vi "HOST_1712.vi"() -> ()   [LabVIEW 2018]
uses:
  <vilib>/userdefined/High Color/nirio_resource_hc.ctl
  <instrlib>/niDCPower/nidcpower.llb/niDCPower Measurement Type.ctl
  <vilib>/FPGAPlugInAG/PXI-7953R/niLvFpga_Open_PXI-7953R.vi
  <vilib>/rvi/interface/common/dynamic/niFpgaDynamicAddResources.vi
  <vilib>/FPGAPlugInAG/Dynamic/niLvFpga_Reset_Dynamic.vi
  <vilib>/FPGAPlugInAG/Dynamic/niLvFpga_Run_Dynamic.vi
  <vilib>/Utility/error.llb/Error Cluster From Error Code.vi
  <vilib>/rvi/errors/niLvFpgaAdjustHostInterfaceError.vi
  <vilib>/FPGAPlugInAG/Dynamic/niLvFpga_Close_Dynamic.vi
  <vilib>/rvi/interface/nirviOpenFPGA/nirviOpenFPGA.xnode
  FPGA Bitfiles/1712_FPGATarget_TARGET1712_0YSosfiRP6w.lvbitx
  <vilib>/rvi/interface/nirviMethod/nirviMethod.xnode
  <vilib>/rvi/interface/nirviReadWriteControl/nirviReadWriteControl.xnode
  <vilib>/rvi/interface/nirviCloseFPGA/nirviCloseFPGA.xnode
  NiFpgaLv.dll
  <vilib>/rvi/interface/Simulation/niFpgaSimulationCallBeginRW.vi
  <vilib>/FPGAPlugInAG/Dynamic/niLvFpga_ReadFifo_Dynamic.vi
  <vilib>/rvi/errors/niLvFpgaMergeErrorWithErrorCode.vi
  <vilib>/Analysis/NI_AALPro.lvlib
panel:
  in  "Включаем автоматом?":bool
  out "VDD":i32
  out "PS":i32
  out "ADC":i32
  out "STAB":i32
  out "-15":i32
  out "4V":i32
  out "RD":i32
  out "PH":i32
  out "1V":i32
  out "БД":i32
  out "Эфф. по верт.":dbl
  out "Эфф. по гор.":dbl
  in  "Частота?":enum16{"MIN", "MAX"}(ring)
  out "СКО выхода от выхода":cluster{dbl[], dbl[]}(graph)={[6201.177706552707, 7595.434558404559, 8732.705797720797, 10087.72774928775, 11406.968846153846, 12631.295284900283, 14025.915, 15297.925598290598, 16480.01816239316, 17633.976495726496, 18869.50398860399, 20178.697706552706, 21306.84829059829, 22549.05603988604, 23809.401296296295, 24777.888917378918, 25884.07384615385, 27016.14232193732, 28208.568333333336, 29233.02923076923, 30354.480085470084, 31398.67948717949, 32328.064900284902, 32988.004458689466, 33587.57784900285, 34215.26438746438, 34782.93656695157, 35292.22700854701, 35768.959216524214, 36186.2800997151, 36566.8903988604, 36910.31642450143, 37239.01190883191, 37548.589829059834, 37829.74592592593, 38094.46146723647, 38321.56247863248, 38509.039344729346, 38634.09653846154, 38688.332564102566], [1408.2462455537227, 1276.6738405632493, 1421.2168940467238, 1726.6350596022562, 1769.1841993647113, 2160.503960124062, 2252.79189873594, 2374.7481159835115, 2690.694572350192, 2422.9048269586224, 2894.1814706198184, 3106.4349457710996, 3064.1792073843126, 3174.8802855895538, 3734.0833095929265, 4280.53840903318, 5096.146959046002, 5242.581747893684, 5382.248367652099, 5356.227733206448, 5575.580587757664, 5438.475052707056, 5246.7833296664485, 6997.312064633342, 6766.519928378316, 6762.928043979101, 6915.84030212127, 7792.281989480644, 8321.967233913709, 8296.431780392239, 10049.627295205792, 10386.237369576253, 10672.701676543498, 9213.355750556748, 9682.971733830318, 9250.473172388141, 10253.422148829253, 9607.6837198, 10679.138619744117, 10335.552449343717]}
  in  "Усреднение":i32=2
  out "Ке":dbl
  in  "Какая фотка?":string
  in  "НЕПРЕРЫВНО":bool
  out "СКО":dbl
  in  "ISO":dbl=1.0
  out "Среднее":dbl
  out "Фотонная калибровка":cluster{dbl[], dbl[]}(graph)={[6201.177706552707, 7595.434558404559, 8732.705797720797, 10087.72774928775, 11406.968846153846, 12631.295284900283, 14025.915, 15297.925598290598, 16480.01816239316, 17633.976495726496, 18869.50398860399, 20178.697706552706, 21306.84829059829, 22549.05603988604, 23809.401296296295, 24777.888917378918, 25884.07384615385, 27016.14232193732, 28208.568333333336, 29233.02923076923, 30354.480085470084, 31398.67948717949, 32328.064900284902, 32988.004458689466, 33587.57784900285, 34215.26438746438, 34782.93656695157, 35292.22700854701, 35768.959216524214, 36186.2800997151, 36566.8903988604, 36910.31642450143, 37239.01190883191, 37548.589829059834, 37829.74592592593, 38094.46146723647, 38321.56247863248, 38509.039344729346, 38634.09653846154, 38688.332564102566], [1408.2462455537227, 1276.6738405632493, 1421.2168940467238, 1726.6350596022562, 1769.1841993647113, 2160.503960124062, 2252.79189873594, 2374.7481159835115, 2690.694572350192, 2422.9048269586224, 2894.1814706198184, 3106.4349457710996, 3064.1792073843126, 3174.8802855895538, 3734.0833095929265, 4280.53840903318, 5096.146959046002, 5242.581747893684, 5382.248367652099, 5356.227733206448, 5575.580587757664, 5438.475052707056, 5246.7833296664485, 6997.312064633342, 6766.519928378316, 6762.928043979101, 6915.84030212127, 7792.281989480644, 8321.967233913709, 8296.431780392239, 10049.627295205792, 10386.237369576253, 10672.701676543498, 9213.355750556748, 9682.971733830318, 9250.473172388141, 10253.422148829253, 9607.6837198, 10679.138619744117, 10335.552449343717]}
  out "Usat, В":dbl
  out "Ssat, АЦП":dbl
  out "Коэффициент наклона":dbl
  out "Светосигнальная":cluster{u8, "ДИСКРЕТ, мс":u8, dbl[]}(graph)={1, "ДИСКРЕТ, мс"=4, [6201.177706552707, 7595.434558404559, 8732.705797720797, 10087.72774928775, 11406.968846153846, 12631.295284900283, 14025.915, 15297.925598290598, 16480.01816239316, 17633.976495726496, 18869.50398860399, 20178.697706552706, 21306.84829059829, 22549.05603988604, 23809.401296296295, 24777.888917378918, 25884.07384615385, 27016.14232193732, 28208.568333333336, 29233.02923076923, 30354.480085470084, 31398.67948717949, 32328.064900284902, 32988.004458689466, 33587.57784900285, 34215.26438746438, 34782.93656695157, 35292.22700854701, 35768.959216524214, 36186.2800997151, 36566.8903988604, 36910.31642450143, 37239.01190883191, 37548.589829059834, 37829.74592592593, 38094.46146723647, 38321.56247863248, 38509.039344729346, 38634.09653846154, 38688.332564102566]}
  in  "Между кадрами, мс":u8=1
  in  "Кол-во итераций":i32=40
  in  "ПРИМЕЧАНИЕ":string
  in  "Frames":path=path "C:/VPL/LabView_PRJ/DOZOR/1712/FRAMES"
  in  "ДИСКРЕТ, мс":u8=4
  out "FRAME_OK":bool
  in  "Расчет":bool
  in  "Какой канал?":enum16{"OUT1", "OUT2", "OUT4"}(ring)
  in  "+/- OUT2":enum16{"-", "+"}(ring)=enum."+"
  in  "Смещение, до 300_OUT2":dbl
  in  "Усиление (до 6)_OUT2":u8=1
  in  "Запись Кадра":bool
  out "АЦП прошит!":bool
  in  "Усиление (до 6)_OUT4":u8=1
  in  "+/- OUT4":enum16{"-", "+"}(ring)=enum."+"
  in  "Смещение, до 300_OUT4":dbl
  out "Image":T1(plugin-control)
  in  "文韧 世男!":bool
  in  "HIGH":u8=22
  in  "LOW":u8=9
  in  "8":u8=24
  in  "HOR":u16=465
  in  "PH1_1":u8=5
  in  "PH1_2":u8=17
  in  "PH2_1":u8=5
  in  "PH2_2":u8=17
  in  "RG1":u8=5
  in  "RG_2":u8=8
  in  "ADC_1":u8=9
  in  "ADC_2":u8=22
  in  "CDS2_1":u8=5
  in  "CDS2_2":u8=18
  in  "CDS1_1":u8=9
  in  "CDS1_2":u8=14
  in  "PS41_2":u16=710
  in  "PS41_1":u16=30
  in  "PS3_2":u16=843
  in  "PS3_1":u16=435
  in  "PS21_2":u16=573
  in  "PS21_1":u16=165
  in  "PS1_1":u16=300
  in  "PS1_2":u16=980
  in  "1163":u16=1163
  in  "Строка триггер":u16=100
  in  "Сколько строк?":i32=270
  in  "Усиление (до 6)_OUT1":u8=1
  in  "Смещение, до 300_OUT1":dbl
  in  "+/- OUT1":enum16{"-", "+"}(ring)=enum."+"
  in  "2/4 V":enum16{"2V", "4V"}(ring)
  in  "3CH/1CH":enum16{"3CH", "1CH"}(ring)=enum."1CH"
  out "Configuration":bool[](array[boolean])=[FALSE, FALSE, FALSE, TRUE, TRUE, FALSE, TRUE, FALSE, FALSE]
  out "PS":bool
  out "VDD":bool
  out "1V":bool
  out "PH":bool
  out "RD":bool
  out "4V":bool
  out "-15":bool
  in  "0,005":dbl=0.005 format="%#_13g"
  out "STAB":bool
  out "ADC":bool
  in  "Прошить АЦП":bool
  in  "PS_LOW, V":dbl=-8.0 caption="voltage level" format="%_6p"
  in  "PS_LOW_curlim":dbl=0.1 caption="current limit" format="%_6p"
  out "PS_LOW_cur":dbl caption="measurement" format="%_6g"
  in  "ADC, V":dbl=6.0 caption="voltage level" format="%_6p"
  in  "RD, V":dbl=13.0 caption="voltage level" format="%_6p"
  in  "PH_LOW, V":dbl=-3.5 caption="voltage level" format="%_6p"
  in  "VDD, V":dbl=17.0 caption="voltage level" format="%_6p"
  in  "ADC_curlim":dbl=0.2 caption="current limit" format="%_6p"
  in  "STAB_curlim":dbl=0.10000000000000003 caption="current limit" format="%_6p"
  in  "RD_curlim":dbl=0.1 caption="current limit" format="%_6p"
  in  "PH_LOW_curlim":dbl=0.1 caption="current limit" format="%_6p"
  in  "1V_curlim":dbl=0.1 caption="current limit" format="%_6p"
  in  "VDD_curlim":dbl=0.1 caption="current limit" format="%_6p"
  out "ADC_cur":dbl caption="measurement" format="%_6g"
  out "STAB_cur":dbl caption="measurement" format="%_6g"
  out "RD_cur":dbl caption="measurement" format="%_6g"
  out "PH_LOW_cur":dbl caption="measurement" format="%_6g"
  out "1V_cur":dbl caption="measurement" format="%_6g"
  out "VDD_cur":dbl caption="measurement" format="%_6g"
  in  "STAB, V":dbl=15.0 caption="voltage level" format="%_6p"
  in  "1V":dbl=1.0 caption="voltage level" format="%_6p"
  in  "4V":dbl=4.0 caption="voltage level" format="%_6p"
  in  "4V_curlim":dbl=0.1 caption="current limit" format="%_6p"
  out "4V_cur":dbl caption="measurement" format="%_6g"
  in  "-15_curlim":dbl=0.1 caption="current limit" format="%_6p"
  out "-15_cur":dbl caption="measurement" format="%_6g"
  in  "-15, V":dbl=-15.0 caption="voltage level" format="%_6p"
  in  "2":refnum<k15>="PXI1Slot4" caption="instrument handle"
  in  "0":refnum<k15>="PXI1Slot2" caption="instrument handle"
  in  "1":refnum<k15>="PXI1Slot3" caption="instrument handle"
  in  "resource name":T2="PXI1Slot5"
  in  "LOGS":path=path "C:/VPL/LabView_PRJ/DOZOR/1712/LOGS"
  in  "Линейки":bool
  in  "Питание":bool
  in  "Стоп":bool
  out "Номер образца":string="1"
  out "OUT":cluster{u16, u16, u16, u16}[][](array[cluster])
  out "FRAME":u16[][](array[numeric])
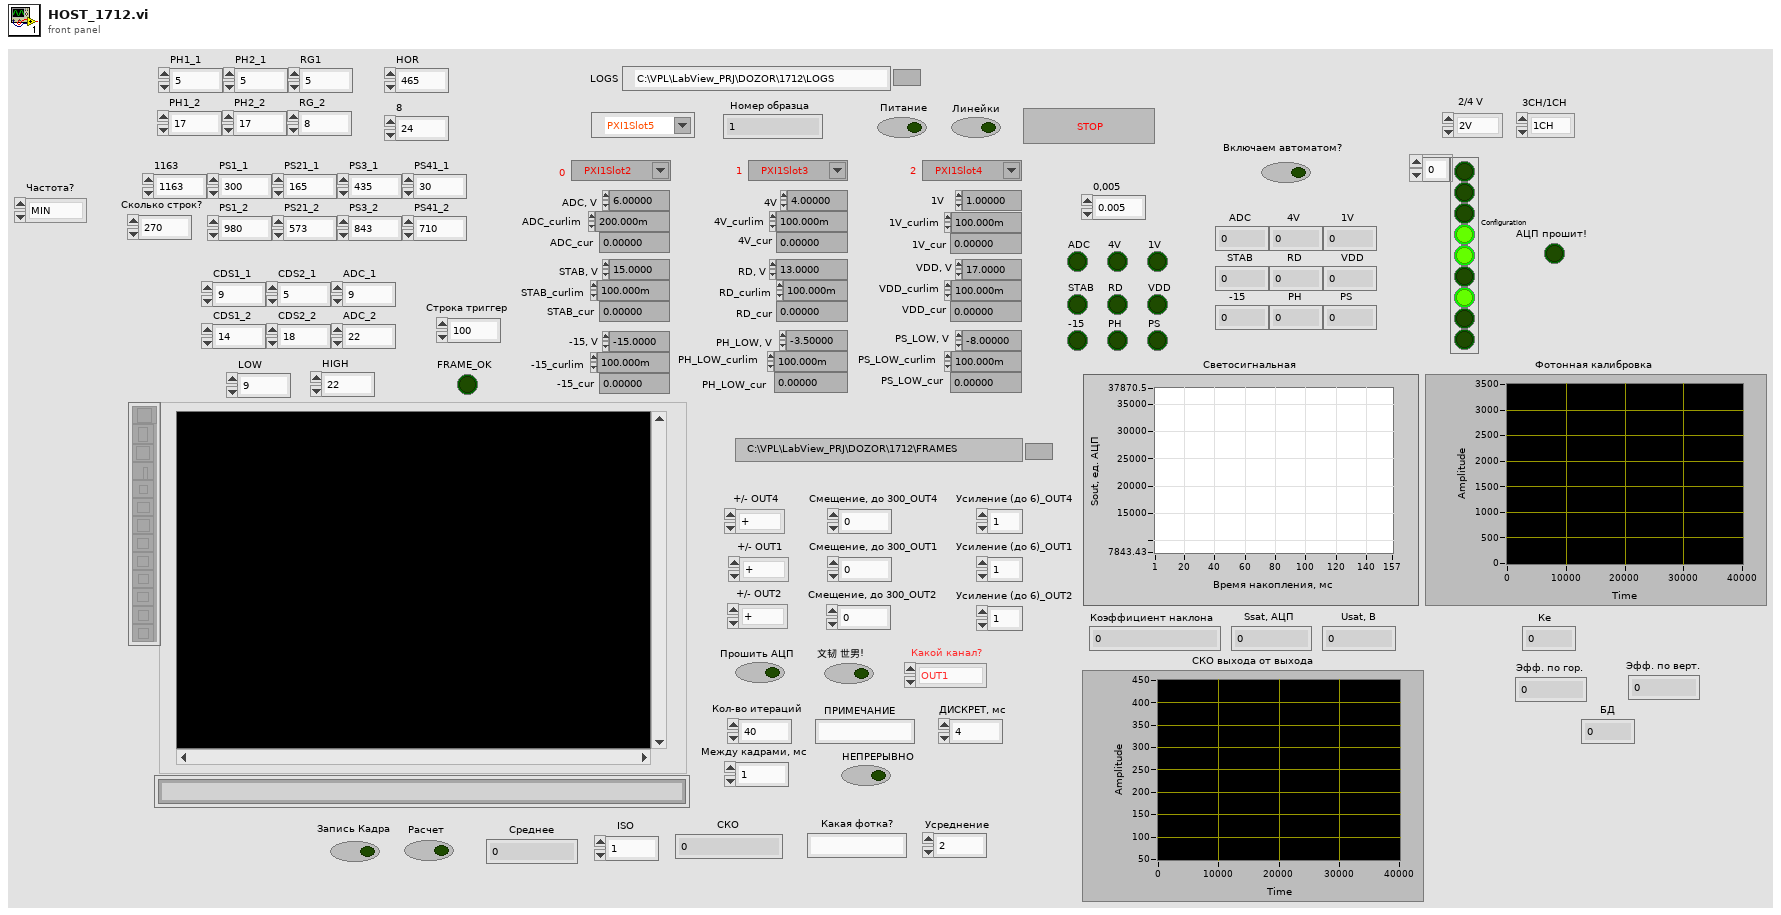
[diagram p1: front panel]
types:
  T1 = typedef "IMAQ Image.ctl" = refnum<image>
  T2 = typedef "nirio_resource_hc.ctl" = tag
  T3 = enum16{"open", "replace", "create", "open or create", "replace or create", "replace or create with confirmation"}
  T4 = typedef "niDCPower Measurement Type.ctl" = i32
  T5 = typedef "Image Type" = u32
  T6 = enum16{"Configuration", "MUX", "RED PGA", "GREEN PGA", "BLUE PGA", "RED OFF", "GREEN OFF", "BLUE OFF"}
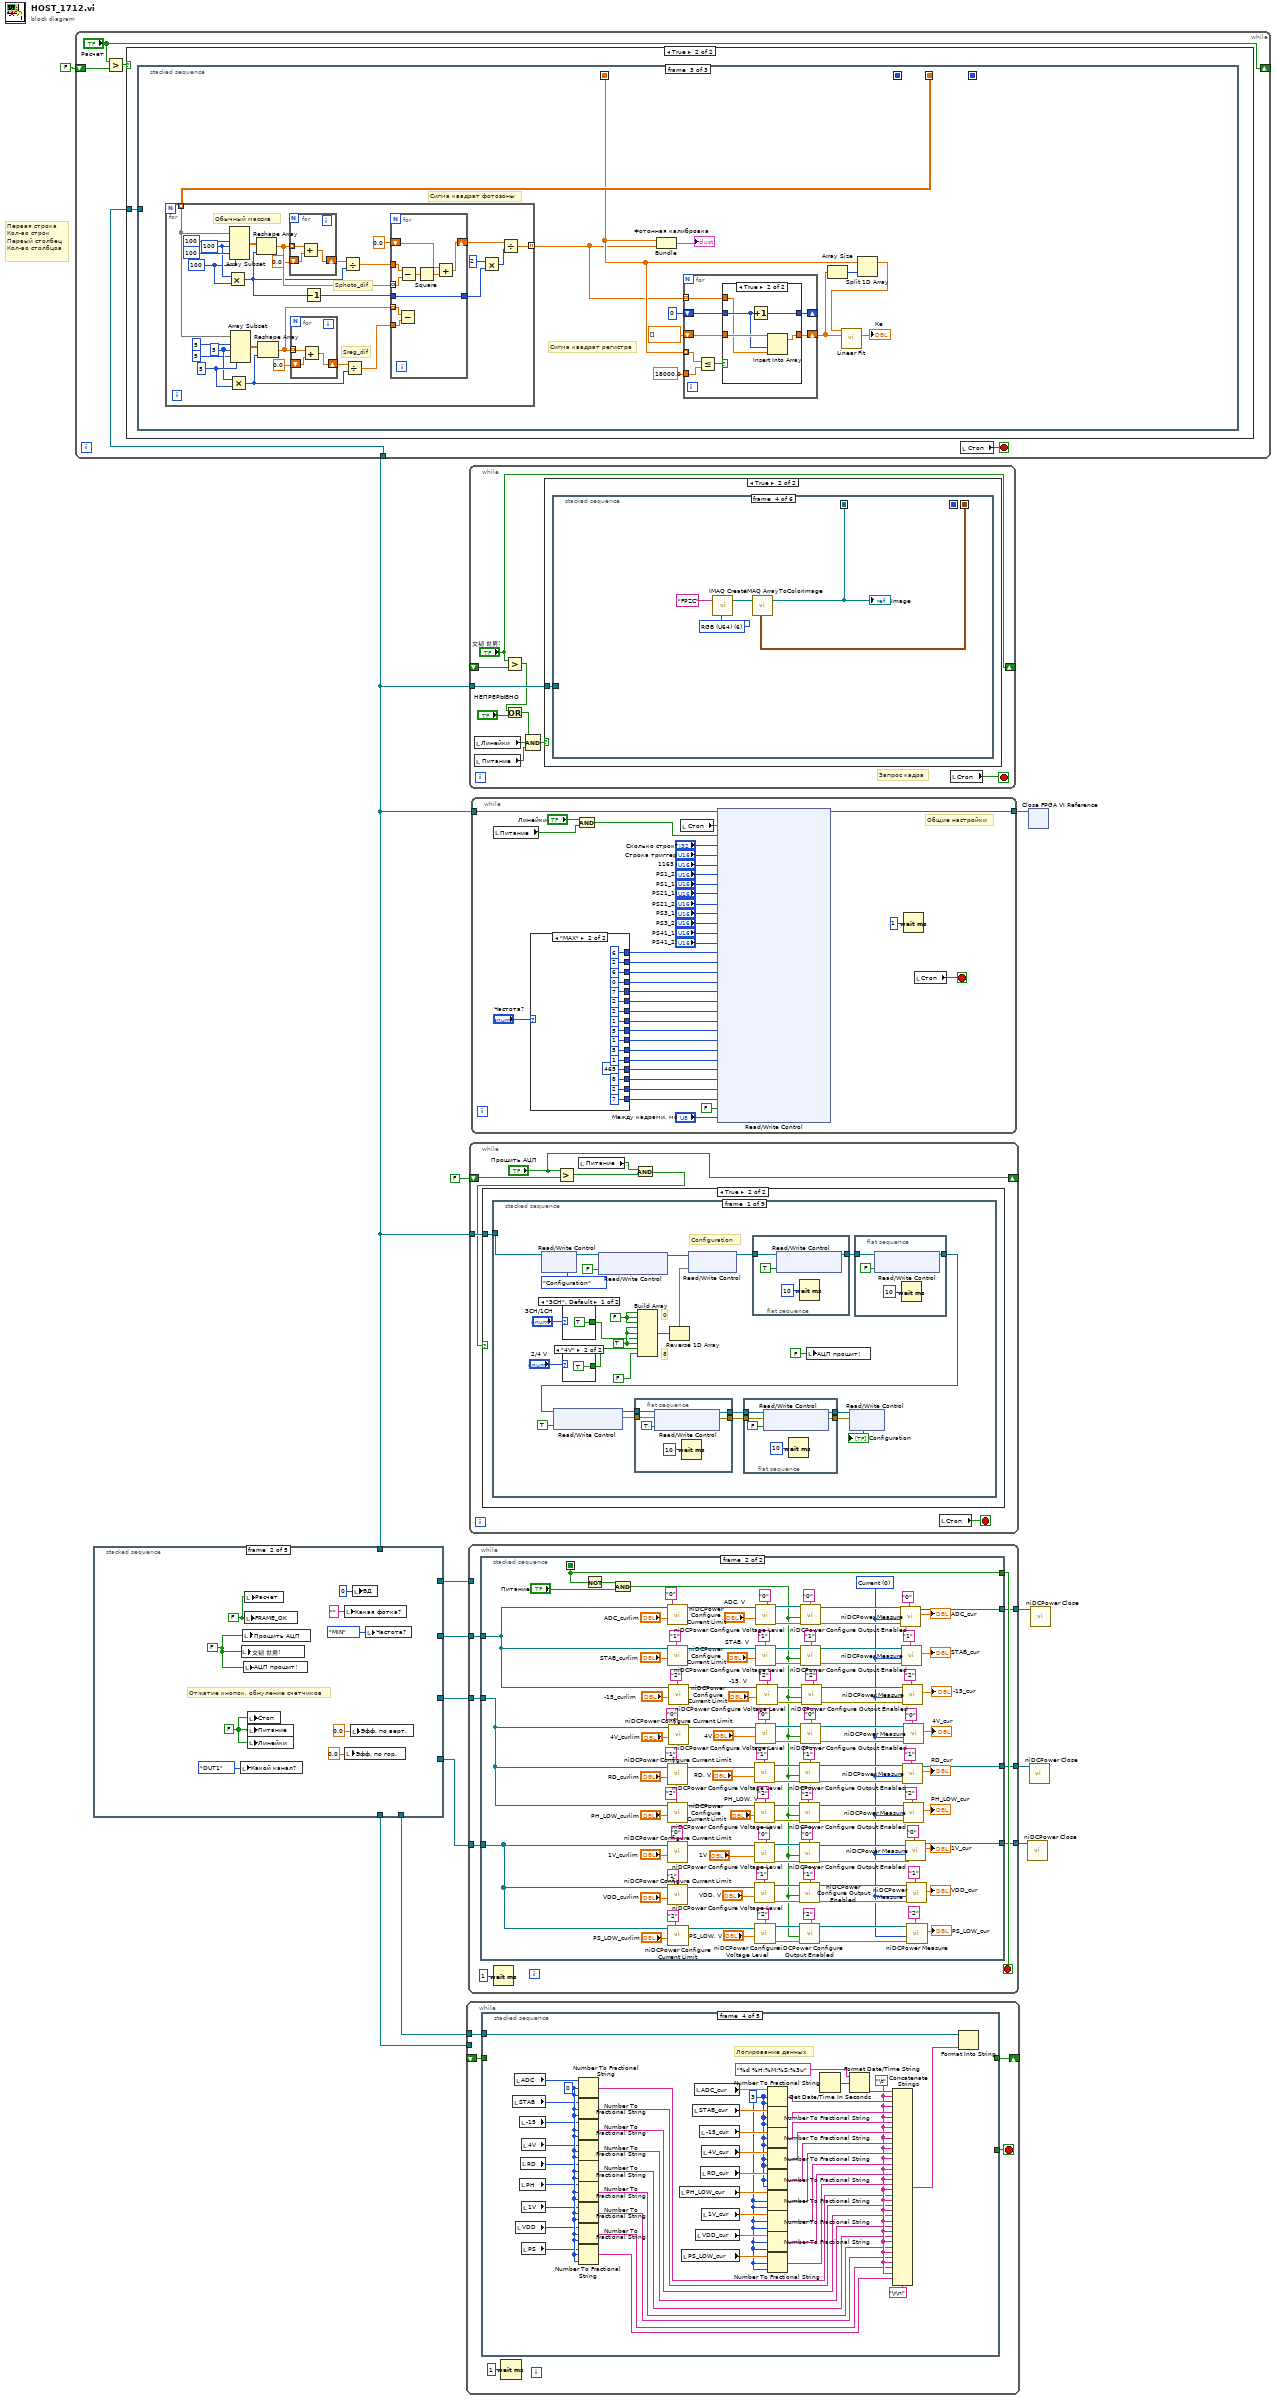
[diagram p0: block diagram]
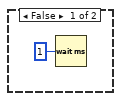
[diagram p2: hidden frame]
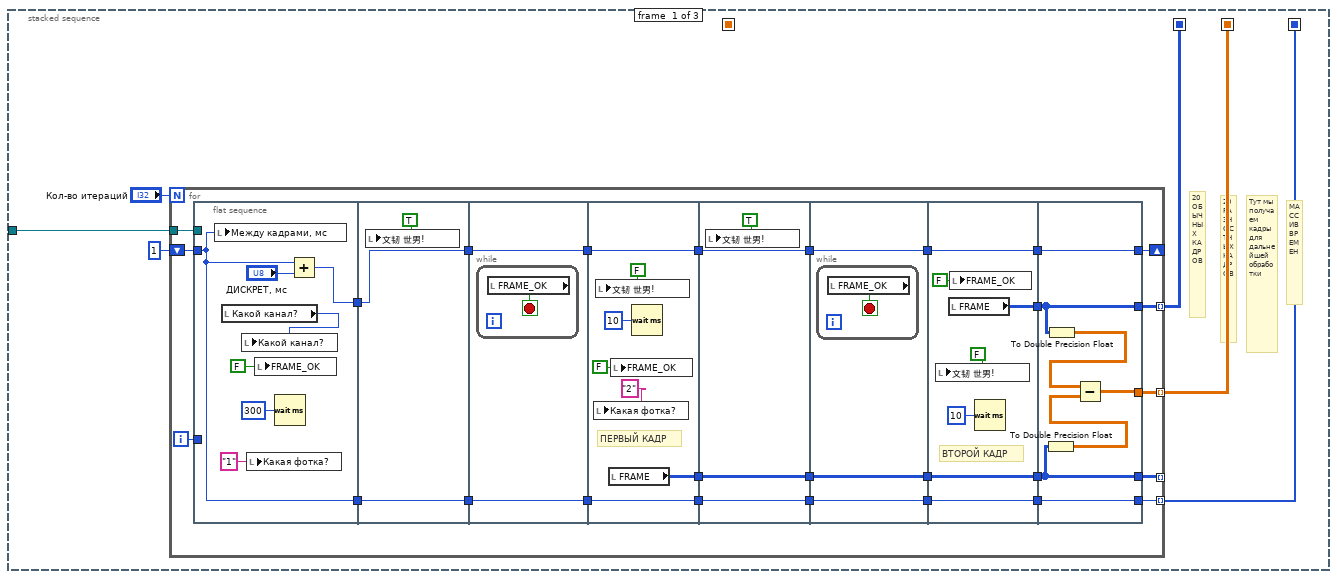
[diagram p3: hidden frame]
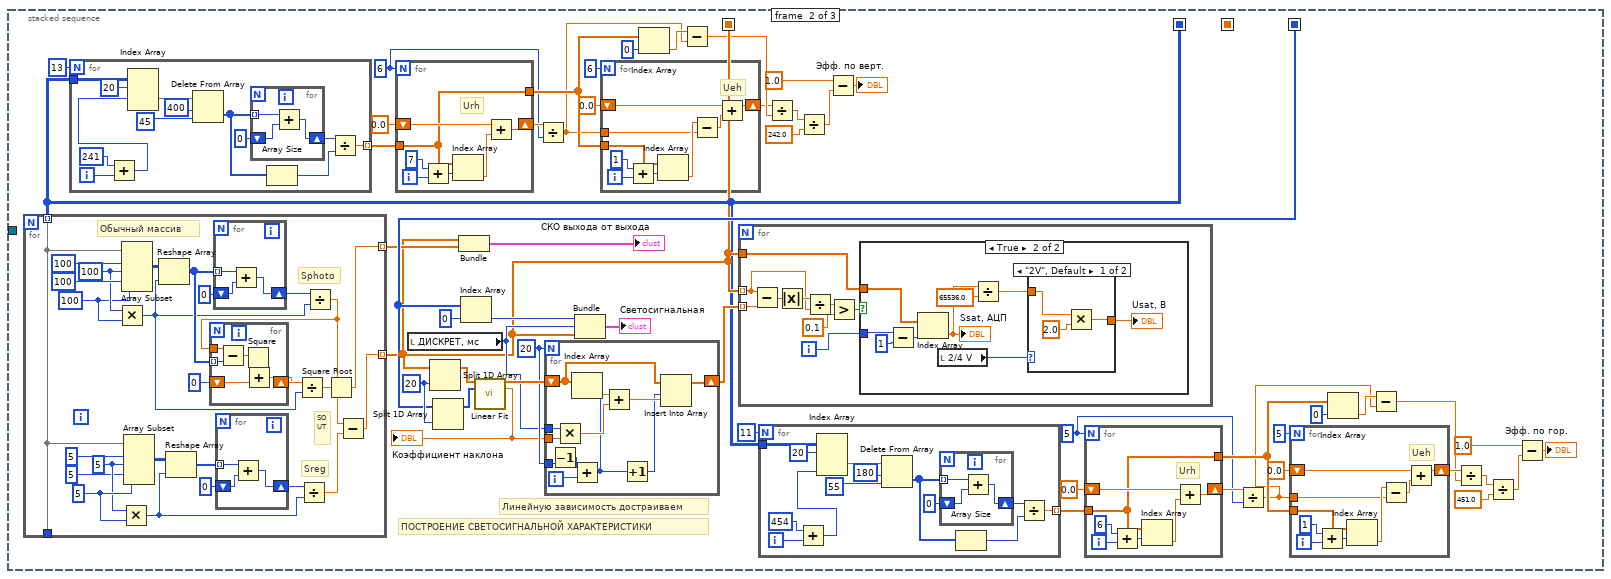
[diagram p4: hidden frame]
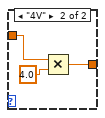
[diagram p6: hidden frame]
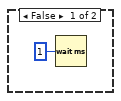
[diagram p8: hidden frame]
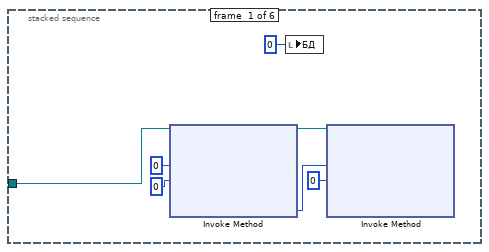
[diagram p9: hidden frame]
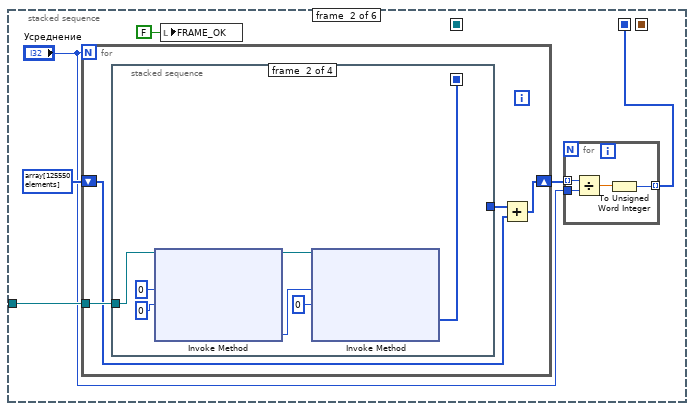
[diagram p10: hidden frame]
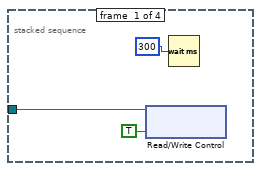
[diagram p11: hidden frame]
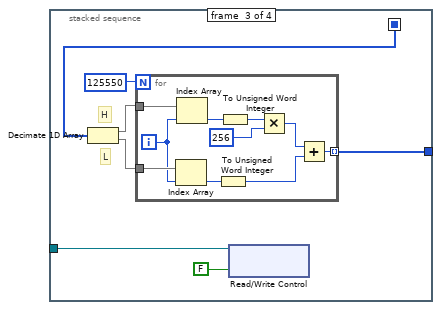
[diagram p12: hidden frame]
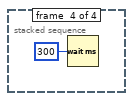
[diagram p13: hidden frame]
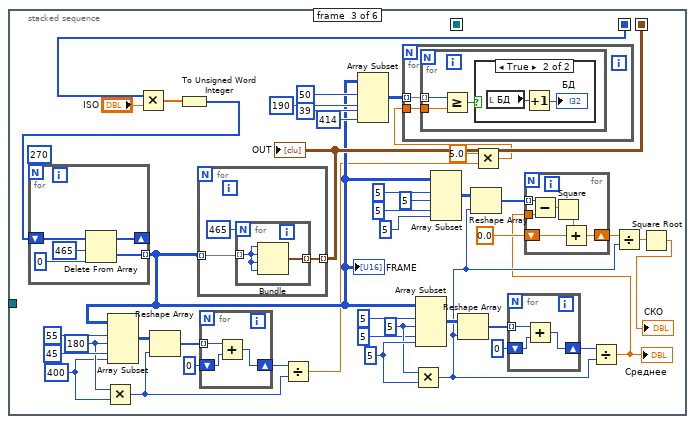
[diagram p14: hidden frame]
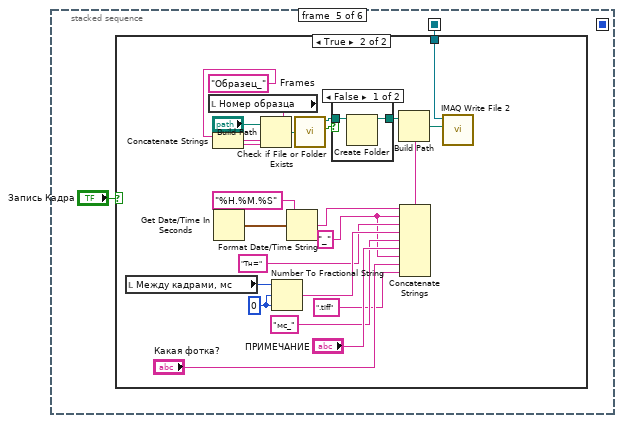
[diagram p16: hidden frame]
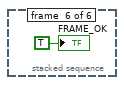
[diagram p19: hidden frame]
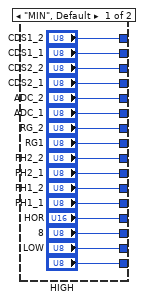
[diagram p20: hidden frame]
diagram:
  # "Первая строка\nКол-во строк\nПервый столбец\nКол-во столбцов"
  n1 = stacked-sequence {
    tunnel: [_ _ _ w61 _] -> w13
    tunnel: [_ _ _ _ w69] -> w10
    tunnel: [_ _ _ _ w68] -> w12
    tunnel: [_ _ _ _ w67] -> w11
    tunnel: [_ _ _ w61 _] -> w1
    tunnel: [_ _ _ w61 _] -> w6
    tunnel: [_ _ w24 _ _] -> w3
    frame #0 {
      n2 = call "Begin.vi"() -> ("Номер образца 2"=→"Номер образца":string)  [unwired: 11 in]
    }
    frame #1 {
      w20 = FALSE ("FRAME_OK")
      w22 = FALSE
      w23 = FALSE ("Стоп")
      # "Отжатие кнопок, обнуление счетчиков"
      n3 = local write "Какой канал?"(enum16{"OUT1", "OUT2", "OUT4"}."OUT1" ("Какой канал?")) -> ()
      n4 = local write "文韧 世男!"(w22) -> ()
      n5 = local write "Прошить АЦП"(w22) -> ()
      n6 = local write "АЦП прошит!"(w22) -> ()
      n7 = local write "FRAME_OK"(w20) -> ()
      n8 = local write "Расчет"(w20) -> ()
      n9 = local write "Стоп"(w23) -> ()
      n10 = local write "Питание"(w23) -> ()
      n11 = local write "Линейки"(w23) -> ()
      n12 = local write "Какая фотка?"("" ("Какая фотка?")) -> ()
      n13 = local write "Эфф. по гор."(0.0 ("Эфф. по гор.")) -> ()
      n14 = local write "Эфф. по верт."(0.0 ("Эфф. по верт.")) -> ()
      n15 = local write "БД"(0 ("БД")) -> ()
      n16 = local write "Частота?"(enum16{"MIN", "MAX"}."MIN" ("Частота?")) -> ()
    }
    frame #2 {
      w26 = "\t"
      n17 = local read "Номер образца"() -> (w53:string)
      n18 = Build Path(base path="LOGS", name or relative path=w53) -> (appended path=w50:path)
      n19 = Get Date/Time In Seconds() -> (seconds since 1Jan1904=w47:timestamp)
      n20 = call <vilib>:"Check if File or Folder Exists.vi"("path"=w50) -> ("file or folder exists?"=w51:bool, "dup path"=w52:path)  [unwired: 8 in, 1 out]
      n21 = Format Date/Time String(time format string (%c)="%d %H.%M.%S", seconds (now)=w47) -> (date/time string=w45:string)  [unwired: 1 in]
      n22 = case shown="False" w51 {
        tunnel: w52 -> [w59 w60]
        tunnel: [w58 w60] -> w42
        frame False {
          n23 = Create Folder(path (use dialog)=w59) -> (created path=w58:path)  [unwired: 2 in, 2 out]
        }
        frame True {
        }
      }
      n24 = Concatenate Strings(w45, ".xls" ("string")) -> (w44:string)
      n25 = Build Path(base path=w42, name or relative path=w44) -> (appended path=w46:path)
      n26 = Open/Create/Replace File(file path (use dialog)=w46, operation (0:open)=T3."open or create", access (0:read/write)=enum16{"read/write", "read-only", "write-only"}."read/write") -> (refnum out=w48:refnum<file>)  [unwired: 3 in, 2 out]
      n27 = case shown="True" TRUE {
        tunnel: w48 -> [w54 w57]
        tunnel: [w54 w55] -> w43
        frame False {
        }
        frame True {
          n28 = Set File Position(refnum=w57, from (0:start)=enum16{"start", "end", "current"}."end") -> (refnum out=w55:refnum<file>)  [unwired: 2 in, 1 out]
        }
      }
      n29 = Format Into String(initial string=w43, "Time" ("input 1"), w26, "ADC_cur", w26, "STAB_cur", w26, "-15_cur", w26, "4_cur", w26, "RD_cur", w26, "PH_LOW_cur", w26, "1V_cur", w26, "VDD_cur", w26, "PS_LOW_cur", "\r\n") -> (resulting string=w24:refnum<file>)  [unwired: 2 in, 1 out]
    }
    frame #3 {
      n30 = xnode "Open FPGA VI Reference"("resource name"="resource name") -> ("FPGA VI Reference Out"=w62:refnum<k20>, "error out"=w64:errorcluster)  [unwired: 1 in]
      n31 = xnode "Invoke Method"("FPGA VI Reference In"=w62, "error in"=w64) -> ("FPGA VI Reference Out"=w65:refnum<k20>, "error out"=w63:errorcluster)
      n32 = xnode "Invoke Method"("FPGA VI Reference In"=w65, "error in"=w63) -> ("FPGA VI Reference Out"=w61:refnum<k20>)  [unwired: 1 in, 1 out]
    }
    frame #4 {
      n33 = call <instrlib>:"niDCPower Initialize.vi"("resource name"="2") -> ("error out"=w75:errorcluster, "instrument handle out"=w72:refnum<k15>)  [unwired: 3 in, 6 out]
      n34 = call <instrlib>:"niDCPower Initialize.vi"("resource name"="1") -> ("error out"=w73:errorcluster, "instrument handle out"=w70:refnum<k15>)  [unwired: 3 in, 6 out]
      n35 = call <instrlib>:"niDCPower Initialize.vi"("resource name"="0") -> ("error out"=w74:errorcluster, "instrument handle out"=w71:refnum<k15>)  [unwired: 3 in, 6 out]
      n36 = call <instrlib>:"niDCPower Configure Voltage Level.vi"("error in (no error)"=w75, "voltage level"=0.0, "channel name"="0,1,2", "instrument handle"=w72) -> ("instrument handle out"=w69:refnum<k15>)  [unwired: 6 in, 1 out]
      n37 = call <instrlib>:"niDCPower Configure Voltage Level.vi"("error in (no error)"=w73, "voltage level"=0.0, "channel name"="0,1,2", "instrument handle"=w70) -> ("instrument handle out"=w67:refnum<k15>)  [unwired: 6 in, 1 out]
      n38 = call <instrlib>:"niDCPower Configure Voltage Level.vi"("error in (no error)"=w74, "voltage level"=0.0, "channel name"="0,1,2", "instrument handle"=w71) -> ("instrument handle out"=w68:refnum<k15>)  [unwired: 6 in, 1 out]
    }
  }
  n39 = while {
    shift-right: ["Расчет"] -> _
    shift-left: FALSE ("Расчет") -> [w87]
    tunnel: w1 -> [w85]
    stop <- w89 stop-if-true
    n40 = Greater?(x="Расчет", y=w87) -> (0:w88:bool)
    n41 = case shown="True" w88 {
      tunnel: w85 -> [_ w91]
      frame False {
        n42 = Wait (ms)(milliseconds to wait=u32 1) -> ()  [unwired: 1 out]
      }
      frame True {
        n43 = stacked-sequence {
          seq-local: [w92 _ _] -> [_ w167 _]
          seq-local: [w94 _ _] -> [_ _ w367]
          seq-local: [w93 _ _] -> [_ w209 _]
          seq-local: [_ w204 _] -> [_ _ w359]
          tunnel: w91 -> [w97 _ _]
          frame #0 {
            # "МАССИВ ВРЕМЕН"
            # "Тут мы получаем кадры\nдля дальнейшей обработки"
            # "20 РАЗНОСТНЫХ КАДРОВ"
            # "20 ОБЫЧНЫХ КАДРОВ"
            n44 = for {
              N: "Кол-во итераций" -> [_]
              tunnel: w97 -> [w124]
              shift-right: [w122] -> _
              shift-left: u8 1 -> [w123]
              tunnel: [w109] -> w92 mode=indexing
              tunnel: [w108] -> w94 mode=indexing
              tunnel: [w107] -> w93 mode=indexing
              tunnel: [w98] -> _ mode=indexing
              i -> [w99]
              n45 = flat-sequence {
                tunnel: w124 -> [_]
                tunnel: w123 -> [w127]
                tunnel: [w130] -> w119
                tunnel: [w127] -> w100
                tunnel: w99 -> [_]
                tunnel: [w134] -> w121
                tunnel: w119 -> [w134]
                tunnel: [w132] -> w101
                tunnel: w100 -> [w132]
                tunnel: w121 -> [w136]
                tunnel: [w136] -> w120
                tunnel: [w135] -> w102
                tunnel: w101 -> [w135]
                tunnel: w120 -> [w144]
                tunnel: [w144] -> w118
                tunnel: [w141] -> w110
                tunnel: [w139] -> w103
                tunnel: w102 -> [w139]
                tunnel: w118 -> [w148]
                tunnel: [w148] -> w117
                tunnel: [w146] -> w111
                tunnel: w110 -> [w146]
                tunnel: [w145] -> w104
                tunnel: w103 -> [w145]
                tunnel: w117 -> [w151]
                tunnel: [w151] -> w116
                tunnel: [w150] -> w112
                tunnel: w111 -> [w150]
                tunnel: [w149] -> w105
                tunnel: w104 -> [w149]
                tunnel: w116 -> [w159]
                tunnel: [w159] -> w115
                tunnel: [w158] -> w114
                tunnel: [w157] -> w113
                tunnel: w112 -> [w157]
                tunnel: [w153] -> w106
                tunnel: w105 -> [w153]
                tunnel: [w166] -> w122
                tunnel: w115 -> [w166]
                tunnel: w114 -> [w164]
                tunnel: w113 -> [w160]
                tunnel: [w163] -> w108
                tunnel: [w164] -> w109
                tunnel: [w165] -> w107
                tunnel: w106 -> [w165]
                tunnel: [w160] -> w98
                frame #0 {
                  n46 = local write "Между кадрами, мс"(w127) -> ()
                  n47 = local read "Какой канал?"() -> (w126:enum16{"OUT1", "OUT2", "OUT4"})
                  n48 = local write "Какой канал?"(w126) -> ()
                  n49 = local write "Какая фотка?"("1" ("Какая фотка?")) -> ()
                  n50 = local write "FRAME_OK"(FALSE ("FRAME_OK")) -> ()
                  n51 = Wait (ms)(milliseconds to wait=u32 300) -> ()  [unwired: 1 out]
                  n52 = Add(x=w127, y="ДИСКРЕТ, мс") -> (x+y=w130:u8)
                }
                frame #1 {
                  n53 = local write "文韧 世男!"(TRUE ("文韧 世男!")) -> ()
                }
                frame #2 {
                  n54 = while {
                    stop <- w137 stop-if-true
                    n55 = local read "FRAME_OK"() -> (w137:bool)
                  }
                }
                frame #3 {
                  # "ПЕРВЫЙ КАДР"
                  n56 = local write "Какая фотка?"("2" ("Какая фотка?")) -> ()
                  n57 = local write "文韧 世男!"(FALSE ("文韧 世男!")) -> ()
                  n58 = local read "FRAME"() -> (w141:u16[][])
                  n59 = local write "FRAME_OK"(FALSE ("FRAME_OK")) -> ()
                  n60 = Wait (ms)(milliseconds to wait=u32 10) -> ()  [unwired: 1 out]
                }
                frame #4 {
                  n61 = local write "文韧 世男!"(TRUE ("文韧 世男!")) -> ()
                }
                frame #5 {
                  n62 = while {
                    stop <- w152 stop-if-true
                    n63 = local read "FRAME_OK"() -> (w152:bool)
                  }
                }
                frame #6 {
                  # "ВТОРОЙ КАДР"
                  n64 = local write "文韧 世男!"(FALSE ("文韧 世男!")) -> ()
                  n65 = local read "FRAME"() -> (w158:u16[][])
                  n66 = local write "FRAME_OK"(FALSE ("FRAME_OK")) -> ()
                  n67 = Wait (ms)(milliseconds to wait=u32 10) -> ()  [unwired: 1 out]
                }
                frame #7 {
                  n68 = To Double Precision Float(number=w160) -> (double precision float=w161:dbl[][])
                  n69 = To Double Precision Float(number=w164) -> (double precision float=w162:dbl[][])
                  n70 = Subtract(x=w162, y=w161) -> (x-y=w163:dbl[][])
                }
              }
            }
          }
          frame #1 {
            w169 = 6
            w170 = 5
            w212 = 20
            w217 = 20 ("index")
            # "ПОСТРОЕНИЕ СВЕТОСИГНАЛЬНОЙ ХАРАКТЕРИСТИКИ"
            # "Линейную зависимость достраиваем"
            n71 = for {
              tunnel: w167 -> [w319] mode=indexing
              tunnel: [w321] -> w204 mode=indexing
              tunnel: [w325] -> w206 mode=indexing
              tunnel: [w319] -> _
              w332 = 5 ("length")
              w331 = 5 ("length")
              w341 = 100 ("length")
              w342 = 100 ("length")
              # "SOUT"
              # "Sreg"
              # "Sphoto"
              # "Обычный массив"
              n72 = Multiply(x=w342, y=w341) -> (x*y=w323:i32)
              n73 = Multiply(x=w331, y=w332) -> (x*y=w337:i32)
              n74 = Array Subset(array=w319, index (row)=100 ("index"), length (row)=w342, index (col)=100 ("index"), length (col)=w341) -> (w340:u16[][])
              n75 = Array Subset(array=w319, index (row)=5 ("index"), length (row)=w331, index (col)=5 ("index"), length (col)=w332) -> (w333:u16[][])
              n76 = Reshape Array(w340, w323) -> (w327:u16[])
              n77 = Reshape Array(w333, w337) -> (w334:u16[])
              n78 = for {
                tunnel: w327 -> [w356] mode=indexing
                shift-right: [w354] -> w338
                shift-left: u64 0 -> [w355]
                n79 = Add(x=w356, y=w355) -> (x+y=w354:u64)
              }
              n80 = for {
                tunnel: w334 -> [w353] mode=indexing
                shift-right: [w351] -> w336
                shift-left: u64 0 -> [w352]
                n81 = Add(x=w353, y=w352) -> (x+y=w351:u64)
              }
              n82 = Divide(x=w336, y=w337) -> (x/y=w328:dbl)
              n83 = Divide(x=w338, y=w323) -> (x/y=w320:dbl)
              n84 = for {
                tunnel: w327 -> [w350] mode=indexing
                shift-right: [w349] -> w324
                shift-left: u64 0 -> [w346]
                tunnel: w320 -> [w345]
                n85 = Subtract(x=w345, y=w350) -> (x-y=w348:dbl)
                n86 = Square(x=w348) -> (x^2=w347:dbl)
                n87 = Add(x=w347, y=w346) -> (x+y=w349:dbl)
              }
              n88 = Divide(x=w324, y=w323) -> (x/y=w322:dbl)
              n89 = Square Root(x=w322) -> (sqrt(x)=w325:dbl)
              n90 = Subtract(x=w320, y=w328) -> (x-y=w321:dbl)
            }
            n91 = for {
              N: 13 -> [_]
              tunnel: w167 -> [w247]
              tunnel: [w236] -> w176 mode=indexing
              i -> [w238]
              n92 = Add(x=241, y=w238) -> (x+y=w235:i32)
              n93 = Index Array(array=w247, index (dim 0)=20 ("disabled index (page)"), index (dim 1)=w235) -> (element=w245:u16[])  [unwired: 1 in]
              n94 = Delete From Array(array=w245, length=400, index=45) -> (deleted portion=w240:u16[])  [unwired: 1 out]
              n95 = for {
                tunnel: w240 -> [w250] mode=indexing
                shift-right: [w248] -> w241
                shift-left: 0 -> [w249]
                n96 = Add(x=w250, y=w249) -> (x+y=w248:i32)
              }
              n97 = Array Size(array=w240) -> (size(s)=w239:i32)
              n98 = Divide(x=w241, y=w239) -> (x/y=w236:dbl)
            }
            n99 = for {
              N: w169 -> [_]
              tunnel: w176 -> [w228]
              shift-right: [w229] -> w172
              shift-left: 0.0 -> [w231]
              tunnel: [w228] -> w181
              i -> [w234]
              # "Urh"
              n100 = Add(x=7, y=w234) -> (x+y=w232:i32)
              n101 = Index Array(array=w228, index=w232) -> (element=w230:dbl)
              n102 = Add(x=w231, y=w230) -> (x+y=w229:dbl)
            }
            n103 = local read "ДИСКРЕТ, мс"() -> (w210:u8)
            n104 = Split 1D Array(array=w204, index=w217) -> (first subarray=w216:dbl[])  [unwired: 1 out]
            n105 = Split 1D Array(array=w209, index=w217) -> (first subarray=w215:u8[])  [unwired: 1 out]
            n106 = Bundle(w204, w206) -> (→"СКО выхода от выхода":cluster{dbl[], dbl[]})  [unwired: 1 in]
            n107 = Index Array(array=w209, index=0) -> (element=w214:u8)
            n108 = call <vilib>:"Linear Fit.vi"("Y"=w216, "X"=w215) -> ("Best Linear Fit"=w213:dbl[], "slope"=w211:dbl)  [unwired: 9 in, 3 out]
            "Коэффициент наклона" <- w211
            n109 = Divide(x=w172, y=w169) -> (x/y=w168:dbl)
            n110 = for {
              N: w212 -> [_]
              tunnel: w212 -> [w308]
              shift-right: [w316] -> w208
              shift-left: w213 -> [w309]
              tunnel: w211 -> [w315]
              tunnel: w210 -> [w314]
              i -> [w318]
              n111 = Decrement(x=w308) -> (x-1=w307:i32)
              n112 = Multiply(x=w314, y=w315) -> (x*y=w313:dbl)
              n113 = Add(x=w307, y=w318) -> (x+y=w311:i32)
              n114 = Index Array(array=w309, index=w311) -> (element=w317:dbl)
              n115 = Add(x=w317, y=w313) -> (x+y=w312:dbl)
              n116 = Increment(x=w311) -> (x+1=w310:i32)
              n117 = Insert Into Array(array=w309, index=w310, new element=w312) -> (w316:dbl[])
            }
            n118 = Bundle(w214, "ДИСКРЕТ, мс"=w210, w204) -> (→"Светосигнальная":cluster{u8, "ДИСКРЕТ, мс":u8, dbl[]})  [unwired: 1 in]
            n119 = for {
              N: 6 -> [_]
              tunnel: w181 -> [w224]
              shift-right: [w219] -> w179
              shift-left: 0.0 -> [w220]
              tunnel: w168 -> [w222]
              i -> [w227]
              # "Ueh"
              n120 = Add(x=1, y=w227) -> (x+y=w225:i32)
              n121 = Index Array(array=w224, index=w225) -> (element=w223:dbl)
              n122 = Subtract(x=w223, y=w222) -> (x-y=w221:dbl)
              n123 = Add(x=w220, y=w221) -> (x+y=w219:dbl)
            }
            n124 = Index Array(array=w181, index=0) -> (element=w182:dbl)
            n125 = Subtract(x=w182, y=w168) -> (x-y=w183:dbl)
            n126 = for {
              tunnel: w204 -> [w283] mode=indexing
              tunnel: w208 -> [w291] mode=indexing
              tunnel: w204 -> [w286]
              i -> [w287]
              n127 = Subtract(x=w283, y=w291) -> (x-y=w284:dbl)
              n128 = Absolute Value(x=w284) -> (abs(x)=w285:dbl)
              n129 = Divide(x=w285, y=w283) -> (x/y=w290:dbl)
              n130 = Greater?(x=w290, y=0.1) -> (0:w288:bool)
              n131 = case shown="True" w288 {
                tunnel: w287 -> [_ w294]
                tunnel: w286 -> [_ w300]
                frame False {
                }
                frame True {
                  n132 = Subtract(x=w294, y=1) -> (x-y=w295:i32)
                  n133 = Index Array(array=w300, index=w295) -> (element=w298:dbl)
                  "Ssat, АЦП" <- w298
                  n134 = local read "2/4 V"() -> (w299:enum16{"2V", "4V"})
                  n135 = Divide(x=w298, y=65536.0) -> (x/y=w296:dbl)
                  n136 = case shown="\"2V\", Default" w299 {
                    tunnel: w296 -> [w302 w306]
                    tunnel: [w301 w304] -> w292
                    frame "2V", Default {
                      n137 = Multiply(x=w302, y=2.0) -> (x*y=w301:dbl)
                    }
                    frame "4V" {
                      n138 = Multiply(x=w306, y=4.0) -> (x*y=w304:dbl)
                    }
                  }
                  "Usat, В" <- w292
                }
              }
            }
            n139 = for {
              N: 11 -> [_]
              tunnel: w167 -> [w279]
              tunnel: [w267] -> w202 mode=indexing
              i -> [w270]
              n140 = Add(x=454, y=w270) -> (x+y=w268:i32)
              n141 = Index Array(array=w279, index (dim 0)=20 ("disabled index (page)"), index (dim 2)=w268) -> (element=w277:u16[])  [unwired: 1 in]
              n142 = Delete From Array(array=w277, length=180, index=55) -> (deleted portion=w272:u16[])  [unwired: 1 out]
              n143 = for {
                tunnel: w272 -> [w282] mode=indexing
                shift-right: [w280] -> w273
                shift-left: 0 -> [w281]
                n144 = Add(x=w282, y=w281) -> (x+y=w280:i32)
              }
              n145 = Array Size(array=w272) -> (size(s)=w271:i32)
              n146 = Divide(x=w273, y=w271) -> (x/y=w267:dbl)
            }
            n147 = Divide(x=w179, y=w183) -> (x/y=w185:dbl)
            n148 = Divide(x=w185, y=242.0) -> (x/y=w187:dbl)
            n149 = Subtract(x=1.0, y=w187) -> (x-y=→"Эфф. по верт.":dbl)
            n150 = for {
              N: w170 -> [_]
              tunnel: w202 -> [w260]
              shift-right: [w261] -> w195
              shift-left: 0.0 -> [w263]
              tunnel: [w260] -> w197
              i -> [w266]
              # "Urh"
              n151 = Add(x=6, y=w266) -> (x+y=w264:i32)
              n152 = Index Array(array=w260, index=w264) -> (element=w262:dbl)
              n153 = Add(x=w263, y=w262) -> (x+y=w261:dbl)
            }
            n154 = Divide(x=w195, y=w170) -> (x/y=w171:dbl)
            n155 = for {
              N: 5 -> [_]
              tunnel: w197 -> [w256]
              shift-right: [w251] -> w199
              shift-left: 0.0 -> [w252]
              tunnel: w171 -> [w254]
              i -> [w259]
              # "Ueh"
              n156 = Add(x=1, y=w259) -> (x+y=w257:i32)
              n157 = Index Array(array=w256, index=w257) -> (element=w255:dbl)
              n158 = Subtract(x=w255, y=w254) -> (x-y=w253:dbl)
              n159 = Add(x=w252, y=w253) -> (x+y=w251:dbl)
            }
            n160 = Index Array(array=w197, index=0) -> (element=w196:dbl)
            n161 = Subtract(x=w196, y=w171) -> (x-y=w194:dbl)
            n162 = Divide(x=w199, y=w194) -> (x/y=w192:dbl)
            n163 = Divide(x=w192, y=451.0) -> (x/y=w190:dbl)
            n164 = Subtract(x=1.0, y=w190) -> (x-y=→"Эфф. по гор.":dbl)
          }
          frame #2 {
            # "Сигма квадрат регистра"
            # "Сигма квадрат фотозоны"
            n165 = for {
              tunnel: w367 -> [w398] mode=indexing
              tunnel: [w387] -> w358 mode=indexing
              w402 = 5 ("length")
              w401 = 5 ("length")
              w407 = 100 ("length")
              w408 = 100 ("length")
              # "Sreg_dif"
              # "Sphoto_dif"
              # "Обычный массив"
              n166 = Multiply(x=w408, y=w407) -> (x*y=w393:i32)
              n167 = Multiply(x=w401, y=w402) -> (x*y=w391:i32)
              n168 = Array Subset(array=w398, index (row)=100 ("index"), length (row)=w408, index (col)=100 ("index"), length (col)=w407) -> (w406:dbl[][])
              n169 = Array Subset(array=w398, index (row)=5 ("index"), length (row)=w401, index (col)=5 ("index"), length (col)=w402) -> (w403:dbl[][])
              n170 = Reshape Array(w406, w393) -> (w396:dbl[])
              n171 = Reshape Array(w403, w391) -> (w395:dbl[])
              n172 = for {
                tunnel: w396 -> [w425] mode=indexing
                shift-right: [w423] -> w405
                shift-left: 0.0 -> [w424]
                n173 = Add(x=w425, y=w424) -> (x+y=w423:dbl)
              }
              n174 = for {
                tunnel: w395 -> [w422] mode=indexing
                shift-right: [w420] -> w404
                shift-left: 0.0 -> [w421]
                n175 = Add(x=w422, y=w421) -> (x+y=w420:dbl)
              }
              n176 = Decrement(x=w393) -> (x-1=w392:i32)
              n177 = Divide(x=w405, y=w393) -> (x/y=w386:dbl)
              n178 = Divide(x=w404, y=w391) -> (x/y=w397:dbl)
              n179 = for {
                tunnel: w386 -> [w417]
                tunnel: w397 -> [w418]
                tunnel: w396 -> [w416] mode=indexing
                tunnel: w395 -> [w419] mode=indexing
                shift-right: [w412] -> w394
                shift-left: 0.0 -> [w413]
                tunnel: [w411] -> w388
                tunnel: w392 -> [w411]
                n180 = Subtract(x=w419, y=w418) -> ()  [unwired: 1 out]
                n181 = Subtract(x=w417, y=w416) -> (x-y=w415:dbl)
                n182 = Square(x=w415) -> (x^2=w414:dbl)
                n183 = Add(x=w413, y=w414) -> (x+y=w412:dbl)
              }
              n184 = Multiply(x=2, y=w388) -> (x*y=w389:i32)
              n185 = Divide(x=w394, y=w389) -> (x/y=w387:dbl)
            }
            n186 = Bundle(w359, w358) -> (→"Фотонная калибровка":cluster{dbl[], dbl[]})  [unwired: 1 in]
            n187 = for {
              tunnel: w359 -> [w373] mode=indexing
              tunnel: 18000.0 -> [w375]
              shift-right: [w369] -> w364
              shift-left: dbl[] [] -> [w372]
              shift-right: [w370] -> _
              shift-left: 0 -> [w371]
              tunnel: w358 -> [w368] mode=indexing
              n188 = Less Or Equal?(x=w373, y=w375) -> (x <= y?=w374:bool)
              n189 = case shown="True" w374 {
                tunnel: w372 -> [w376 w382]
                tunnel: w371 -> [w377 w380]
                tunnel: [w377 w381] -> w370
                tunnel: [w376 w379] -> w369
                tunnel: w368 -> [_ w378]
                frame False {
                }
                frame True {
                  n190 = Increment(x=w380) -> (x+1=w381:i32)
                  n191 = Insert Into Array(array=w382, index=w380, new element=w378) -> (w379:dbl[])
                }
              }
            }
            n192 = Array Size(array=w364) -> (size(s)=w363:i32)
            n193 = Split 1D Array(array=w359, index=w363) -> (first subarray=w362:dbl[])  [unwired: 1 out]
            n194 = call <vilib>:"Linear Fit.vi"("Y"=w362, "X"=w364) -> ("slope"=→"Ке":dbl)  [unwired: 9 in, 4 out]
          }
        }
      }
    }
    n195 = local read "Стоп"() -> (w89:bool)
  }
  n196 = while {
    shift-right: [w428] -> _
    shift-left: _ -> [w429]
    tunnel: w6 -> [_]
    tunnel: w3 -> [w426]
    stop <- w427 stop-if-true
    n197 = stacked-sequence {
      tunnel: [_ _ _ _ w551] -> w427
      tunnel: w429 -> [w433 _ _ _ _]
      tunnel: [w432 _ _ _ _] -> w428
      tunnel: w426 -> [_ _ _ w527 _]
      frame #0 {
        n198 = local read "Питание"() -> (w432:bool)
        n199 = Greater?(x=w432, y=w433) -> (0:w431:bool)
        n200 = case shown="True" w431 {
          frame False {
          }
          frame True {
            n201 = flat-sequence {
              frame #0 {
                n202 = Wait (ms)(milliseconds to wait=u32 500) -> ()  [unwired: 1 out]
              }
              frame #1 {
                n203 = local write "Прошить АЦП"(TRUE ("Прошить АЦП")) -> ()
                n204 = Wait (ms)(milliseconds to wait=u32 25) -> ()  [unwired: 1 out]
              }
              frame #2 {
                n205 = local write "Прошить АЦП"(FALSE ("Прошить АЦП")) -> ()
                n206 = Wait (ms)(milliseconds to wait=u32 25) -> ()  [unwired: 1 out]
              }
            }
          }
        }
      }
      frame #1 {
        n207 = local read "Питание"() -> (w439:bool)
        n208 = case shown="True" w439 {
          frame False {
          }
          frame True {
            n209 = local read "1V_cur"() -> (w449:dbl)
            n210 = local read "1V_curlim"() -> (w448:dbl)
            n211 = local read "0,005"() -> (w443:dbl)
            n212 = local read "4V_curlim"() -> (w464:dbl)
            n213 = local read "ADC_cur"() -> (w478:dbl)
            n214 = local read "ADC_curlim"() -> (w477:dbl)
            n215 = local read "0,005"() -> (w454:dbl)
            n216 = local read "4V_cur"() -> (w465:dbl)
            n217 = Subtract(x=w464, y=w454) -> (x-y=w466:dbl)
            n218 = Subtract(x=w448, y=w443) -> (x-y=w452:dbl)
            n219 = Subtract(x=w477, y="0,005") -> (x-y=w476:dbl)
            n220 = Greater?(x=w465, y=w466) -> (0:→"4V":bool)
            n221 = Greater?(x=w449, y=w452) -> (0:→"1V":bool)
            n222 = Greater?(x=w478, y=w476) -> (0:→"ADC":bool)
            n223 = local read "RD_curlim"() -> (w461:dbl)
            n224 = local read "VDD_cur"() -> (w447:dbl)
            n225 = local read "VDD_curlim"() -> (w446:dbl)
            n226 = local read "RD_cur"() -> (w462:dbl)
            n227 = local read "STAB_cur"() -> (w473:dbl)
            n228 = local read "STAB_curlim"() -> (w472:dbl)
            n229 = Subtract(x=w461, y=w454) -> (x-y=w460:dbl)
            n230 = Greater?(x=w462, y=w460) -> (0:→"RD":bool)
            n231 = local read "PH_LOW_curlim"() -> (w455:dbl)
            n232 = Subtract(x=w446, y=w443) -> (x-y=w451:dbl)
            n233 = Subtract(x=w472, y="0,005") -> (x-y=w474:dbl)
            n234 = Greater?(x=w447, y=w451) -> (0:→"VDD":bool)
            n235 = local read "PH_LOW_cur"() -> (w456:dbl)
            n236 = Greater?(x=w473, y=w474) -> (0:→"STAB":bool)
            n237 = local read "-15_curlim"() -> (w468:dbl)
            n238 = local read "PS_LOW_cur"() -> (w445:dbl)
            n239 = local read "PS_LOW_curlim"() -> (w444:dbl)
            n240 = Subtract(x=w455, y=w454) -> (x-y=w457:dbl)
            n241 = local read "-15_cur"() -> (w469:dbl)
            n242 = Greater?(x=w456, y=w457) -> (0:→"PH":bool)
            n243 = Subtract(x=w468, y="0,005") -> (x-y=w470:dbl)
            n244 = Greater?(x=w469, y=w470) -> (0:→"-15":bool)
            n245 = Subtract(x=w444, y=w443) -> (x-y=w450:dbl)
            n246 = Greater?(x=w445, y=w450) -> (0:→"PS":bool)
          }
        }
      }
      frame #2 {
        n247 = local read "ADC"() -> (w481:bool)
        n248 = local read "STAB"() -> (w480:bool)
        n249 = local read "-15"() -> (w479:bool)
        n250 = local read "4V"() -> (w484:bool)
        n251 = local read "VDD"() -> (w483:bool)
        n252 = local read "PS"() -> (w482:bool)
        n253 = case shown="True" w483 {
          frame False {
          }
          frame True {
            n254 = local read "VDD"() -> (w505:i32)
            n255 = Increment(x=w505) -> (x+1=→"VDD":i32)
          }
        }
        n256 = case shown="True" w482 {
          frame False {
          }
          frame True {
            n257 = local read "PS"() -> (w503:i32)
            n258 = Increment(x=w503) -> (x+1=→"PS":i32)
          }
        }
        n259 = case shown="True" w481 {
          frame False {
          }
          frame True {
            n260 = local read "ADC"() -> (w501:i32)
            n261 = Increment(x=w501) -> (x+1=→"ADC":i32)
          }
        }
        n262 = case shown="True" w480 {
          frame False {
          }
          frame True {
            n263 = local read "STAB"() -> (w499:i32)
            n264 = Increment(x=w499) -> (x+1=→"STAB":i32)
          }
        }
        n265 = case shown="True" w479 {
          frame False {
          }
          frame True {
            n266 = local read "-15"() -> (w497:i32)
            n267 = Increment(x=w497) -> (x+1=→"-15":i32)
          }
        }
        n268 = case shown="True" w484 {
          frame False {
          }
          frame True {
            n269 = local read "4V"() -> (w495:i32)
            n270 = Increment(x=w495) -> (x+1=→"4V":i32)
          }
        }
        n271 = local read "RD"() -> (w485:bool)
        n272 = local read "PH"() -> (w486:bool)
        n273 = local read "1V"() -> (w487:bool)
        n274 = case shown="True" w486 {
          frame False {
          }
          frame True {
            n275 = local read "PH"() -> (w491:i32)
            n276 = Increment(x=w491) -> (x+1=→"PH":i32)
          }
        }
        n277 = case shown="True" w485 {
          frame False {
          }
          frame True {
            n278 = local read "RD"() -> (w493:i32)
            n279 = Increment(x=w493) -> (x+1=→"RD":i32)
          }
        }
        n280 = case shown="True" w487 {
          frame False {
          }
          frame True {
            n281 = local read "1V"() -> (w489:i32)
            n282 = Increment(x=w489) -> (x+1=→"1V":i32)
          }
        }
      }
      frame #3 {
        w526 = i16 0 ("width (-)")
        w529 = i16 3 ("width (-)")
        w525 = "\t"
        # "Логирование данных"
        n283 = local read "STAB"() -> (w513:i32)
        n284 = local read "ADC"() -> (w514:i32)
        n285 = local read "VDD"() -> (w507:i32)
        n286 = local read "-15"() -> (w512:i32)
        n287 = local read "PH"() -> (w509:i32)
        n288 = local read "RD"() -> (w510:i32)
        n289 = local read "4V"() -> (w511:i32)
        n290 = local read "1V"() -> (w508:i32)
        n291 = local read "PS"() -> (w506:i32)
        n292 = Number To Fractional String(number=w514, width (-)=w526, precision (6)=w526) -> (F-format string=w523:string)  [unwired: 1 in]
        n293 = Number To Fractional String(number=w513, width (-)=w526, precision (6)=w526) -> (F-format string=w522:string)  [unwired: 1 in]
        n294 = Number To Fractional String(number=w512, width (-)=w526, precision (6)=w526) -> (F-format string=w521:string)  [unwired: 1 in]
        n295 = Number To Fractional String(number=w511, width (-)=w526, precision (6)=w526) -> (F-format string=w520:string)  [unwired: 1 in]
        n296 = Number To Fractional String(number=w510, width (-)=w526, precision (6)=w526) -> (F-format string=w519:string)  [unwired: 1 in]
        n297 = Number To Fractional String(number=w509, width (-)=w526, precision (6)=w526) -> (F-format string=w518:string)  [unwired: 1 in]
        n298 = Number To Fractional String(number=w508, width (-)=w526, precision (6)=w526) -> (F-format string=w517:string)  [unwired: 1 in]
        n299 = Number To Fractional String(number=w507, width (-)=w526, precision (6)=w526) -> (F-format string=w516:string)  [unwired: 1 in]
        n300 = Number To Fractional String(number=w506, width (-)=w526, precision (6)=w526) -> (F-format string=w515:string)  [unwired: 1 in]
        n301 = local read "PH_LOW_cur"() -> (w533:dbl)
        n302 = local read "PS_LOW_cur"() -> (w530:dbl)
        n303 = local read "STAB_cur"() -> (w537:dbl)
        n304 = local read "ADC_cur"() -> (w538:dbl)
        n305 = local read "VDD_cur"() -> (w531:dbl)
        n306 = local read "-15_cur"() -> (w536:dbl)
        n307 = local read "RD_cur"() -> (w534:dbl)
        n308 = local read "4V_cur"() -> (w535:dbl)
        n309 = local read "1V_cur"() -> (w532:dbl)
        n310 = Number To Fractional String(number=w538, width (-)=w529, precision (6)=w529) -> (F-format string=w547:string)  [unwired: 1 in]
        n311 = Number To Fractional String(number=w537, width (-)=w529, precision (6)=w529) -> (F-format string=w546:string)  [unwired: 1 in]
        n312 = Number To Fractional String(number=w536, width (-)=w529, precision (6)=w529) -> (F-format string=w545:string)  [unwired: 1 in]
        n313 = Number To Fractional String(number=w535, width (-)=w529, precision (6)=w529) -> (F-format string=w544:string)  [unwired: 1 in]
        n314 = Number To Fractional String(number=w534, width (-)=w529, precision (6)=w529) -> (F-format string=w543:string)  [unwired: 1 in]
        n315 = Number To Fractional String(number=w533, width (-)=w529, precision (6)=w529) -> (F-format string=w542:string)  [unwired: 1 in]
        n316 = Number To Fractional String(number=w532, width (-)=w529, precision (6)=w529) -> (F-format string=w541:string)  [unwired: 1 in]
        n317 = Number To Fractional String(number=w531, width (-)=w529, precision (6)=w529) -> (F-format string=w540:string)  [unwired: 1 in]
        n318 = Number To Fractional String(number=w530, width (-)=w529, precision (6)=w529) -> (F-format string=w539:string)  [unwired: 1 in]
        n319 = Get Date/Time In Seconds() -> (seconds since 1Jan1904=w550:timestamp)
        n320 = Format Date/Time String(time format string (%c)="%d %H:%M:%S:%3u", seconds (now)=w550) -> (date/time string=w548:string)  [unwired: 1 in]
        n321 = Concatenate Strings(w548, w525, w547, w525, w546, w525, w545, w525, w544, w525, w543, w525, w542, w525, w541, w525, w540, w525, w539, w525, w523, w525, w522, w525, w521, w525, w520, w525, w519, w525, w518, w525, w517, w525, w516, w525, w515, "\r\n") -> (w549:string)
        n322 = Format Into String(initial string=w527, w549) -> ()  [unwired: 2 in, 2 out]
      }
      frame #4 {
        n323 = flat-sequence {
          frame #0 {
            n324 = local read "STAB"() -> (w558:bool)
            n325 = local read "ADC"() -> (w559:bool)
            n326 = local read "VDD"() -> (w561:bool)
            n327 = local read "-15"() -> (w557:bool)
            n328 = local read "PS"() -> (w560:bool)
            n329 = local read "4V"() -> (w556:bool)
            n330 = local read "RD"() -> (w555:bool)
            n331 = local read "PH"() -> (w554:bool)
            n332 = local read "1V"() -> (w553:bool)
            n333 = Compound Arithmetic op=OR(w561, w560, w559, w558, w557, w556, w555, w554, w553) -> (w552:bool)
            n334 = case shown="True" w552 {
              selector: w552 -> [_ w563]
              frame False {
              }
              frame True {
                n335 = Not(x=w563) -> (.not. x?=w562:bool)
                n336 = local write "Питание"(w562) -> ()
              }
            }
          }
          frame #1 {
            n337 = case shown="True" "Включаем автоматом?" {
              frame False {
              }
              frame True {
                n338 = flat-sequence {
                  frame #0 {
                    n339 = Wait (ms)(milliseconds to wait=u32 100) -> ()  [unwired: 1 out]
                  }
                  frame #1 {
                    n340 = local write "Питание"(TRUE ("Питание")) -> ()
                  }
                  frame #2 {
                    n341 = Wait (ms)(milliseconds to wait=u32 100) -> ()  [unwired: 1 out]
                  }
                }
              }
            }
          }
        }
        n342 = local read "Стоп"() -> (w551:bool)
      }
    }
    n343 = Wait (ms)(milliseconds to wait=u32 1) -> ()  [unwired: 1 out]
  }
  n344 = while {
    tunnel: w13 -> [_]
    tunnel: w12 -> [w574]
    tunnel: w11 -> [w573]
    tunnel: w10 -> [w572]
    tunnel: [w570] -> w9
    tunnel: [w569] -> w8
    tunnel: [w568] -> w7
    stop <- w571 stop-if-true
    n345 = stacked-sequence {
      seq-local: ["Стоп" _] -> [_ w577]
      tunnel: w572 -> [_ w582]
      tunnel: [_ w623] -> w570
      tunnel: [_ w622] -> w569
      tunnel: [_ w621] -> w568
      tunnel: w574 -> [_ w581]
      tunnel: w573 -> [_ w580]
      tunnel: [_ w577] -> w571
      frame #0 {
      }
      frame #1 {
        w583 = T4 0 items=["Current", "Voltage"] ("measurement type")
        n346 = Not(x=w577) -> (.not. x?=w596:bool)
        n347 = And(x=w596, y="Питание") -> (x .and. y?=w578:bool)
        n348 = call <instrlib>:"niDCPower Configure Current Limit.vi"("current limit"="ADC_curlim", "channel name"="0", "instrument handle"=w581) -> ("instrument handle out"=w658:refnum<k15>)  [unwired: 7 in, 1 out]
        n349 = call <instrlib>:"niDCPower Configure Current Limit.vi"("current limit"="STAB_curlim", "channel name"="1", "instrument handle"=w581) -> ("instrument handle out"=w659:refnum<k15>)  [unwired: 7 in, 1 out]
        n350 = call <instrlib>:"niDCPower Configure Current Limit.vi"("current limit"="RD_curlim", "channel name"="1", "instrument handle"=w580) -> ("instrument handle out"=w660:refnum<k15>)  [unwired: 7 in, 1 out]
        n351 = call <instrlib>:"niDCPower Configure Current Limit.vi"("current limit"="PH_LOW_curlim", "channel name"="2", "instrument handle"=w580) -> ("instrument handle out"=w661:refnum<k15>)  [unwired: 7 in, 1 out]
        n352 = call <instrlib>:"niDCPower Configure Current Limit.vi"("current limit"="1V_curlim", "channel name"="0", "instrument handle"=w582) -> ("instrument handle out"=w662:refnum<k15>)  [unwired: 7 in, 1 out]
        n353 = call <instrlib>:"niDCPower Configure Current Limit.vi"("current limit"="VDD_curlim", "channel name"="1", "instrument handle"=w582) -> ("instrument handle out"=w663:refnum<k15>)  [unwired: 7 in, 1 out]
        n354 = call <instrlib>:"niDCPower Configure Current Limit.vi"("current limit"="PS_LOW_curlim", "channel name"="2", "instrument handle"=w582) -> ("instrument handle out"=w589:refnum<k15>)  [unwired: 7 in, 1 out]
        n355 = call <instrlib>:"niDCPower Configure Current Limit.vi"("current limit"="-15_curlim", "channel name"="2", "instrument handle"=w581) -> ("instrument handle out"=w603:refnum<k15>)  [unwired: 7 in, 1 out]
        n356 = call <instrlib>:"niDCPower Configure Current Limit.vi"("current limit"="4V_curlim", "channel name"="0", "instrument handle"=w580) -> ("instrument handle out"=w614:refnum<k15>)  [unwired: 7 in, 1 out]
        n357 = call <instrlib>:"niDCPower Configure Voltage Level.vi"("voltage level"="RD, V", "channel name"="1", "instrument handle"=w660) -> ("error out"=w641:errorcluster, "instrument handle out"=w638:refnum<k15>)  [unwired: 7 in]
        n358 = call <instrlib>:"niDCPower Configure Voltage Level.vi"("voltage level"="PH_LOW, V", "channel name"="2", "instrument handle"=w661) -> ("error out"=w640:errorcluster, "instrument handle out"=w639:refnum<k15>)  [unwired: 7 in]
        n359 = call <instrlib>:"niDCPower Configure Voltage Level.vi"("voltage level"="1V", "channel name"="0", "instrument handle"=w662) -> ("error out"=w650:errorcluster, "instrument handle out"=w653:refnum<k15>)  [unwired: 7 in]
        n360 = call <instrlib>:"niDCPower Configure Voltage Level.vi"("voltage level"="VDD, V", "channel name"="1", "instrument handle"=w663) -> ("error out"=w651:errorcluster, "instrument handle out"=w652:refnum<k15>)  [unwired: 7 in]
        n361 = call <instrlib>:"niDCPower Configure Voltage Level.vi"("voltage level"="PS_LOW, V", "channel name"="2", "instrument handle"=w589) -> ("error out"=w592:errorcluster, "instrument handle out"=w591:refnum<k15>)  [unwired: 7 in]
        n362 = call <instrlib>:"niDCPower Configure Voltage Level.vi"("voltage level"="ADC, V", "channel name"="0", "instrument handle"=w658) -> ("error out"=w628:errorcluster, "instrument handle out"=w631:refnum<k15>)  [unwired: 7 in]
        n363 = call <instrlib>:"niDCPower Configure Voltage Level.vi"("voltage level"="STAB, V", "channel name"="1", "instrument handle"=w659) -> ("error out"=w629:errorcluster, "instrument handle out"=w630:refnum<k15>)  [unwired: 7 in]
        n364 = call <instrlib>:"niDCPower Configure Voltage Level.vi"("voltage level"="4V", "channel name"="0", "instrument handle"=w614) -> ("error out"=w618:errorcluster, "instrument handle out"=w619:refnum<k15>)  [unwired: 7 in]
        n365 = call <instrlib>:"niDCPower Configure Voltage Level.vi"("voltage level"="-15, V", "channel name"="2", "instrument handle"=w603) -> ("error out"=w606:errorcluster, "instrument handle out"=w605:refnum<k15>)  [unwired: 7 in]
        n366 = call <instrlib>:"niDCPower Configure Output Enabled.vi"("error in (no error)"=w641, "output enabled"=w578, "channel name"="1", "instrument handle"=w638) -> ("error out"=w687:errorcluster, "instrument handle out"=w680:refnum<k15>)  [unwired: 6 in]
        n367 = call <instrlib>:"niDCPower Configure Output Enabled.vi"("error in (no error)"=w640, "output enabled"=w578, "channel name"="2", "instrument handle"=w639) -> ("error out"=w682:errorcluster, "instrument handle out"=w681:refnum<k15>)  [unwired: 6 in]
        n368 = call <instrlib>:"niDCPower Configure Output Enabled.vi"("error in (no error)"=w650, "output enabled"=w578, "channel name"="0", "instrument handle"=w653) -> ("error out"=w684:errorcluster, "instrument handle out"=w683:refnum<k15>)  [unwired: 6 in]
        n369 = call <instrlib>:"niDCPower Configure Output Enabled.vi"("error in (no error)"=w651, "output enabled"=w578, "channel name"="1", "instrument handle"=w652) -> ("error out"=w685:errorcluster, "instrument handle out"=w686:refnum<k15>)  [unwired: 6 in]
        n370 = call <instrlib>:"niDCPower Configure Output Enabled.vi"("error in (no error)"=w592, "output enabled"=w578, "channel name"="2", "instrument handle"=w591) -> ("error out"=w586:errorcluster, "instrument handle out"=w585:refnum<k15>)  [unwired: 6 in]
        n371 = call <instrlib>:"niDCPower Configure Output Enabled.vi"("error in (no error)"=w628, "output enabled"=w578, "channel name"="0", "instrument handle"=w631) -> ("error out"=w671:errorcluster, "instrument handle out"=w670:refnum<k15>)  [unwired: 6 in]
        n372 = call <instrlib>:"niDCPower Configure Output Enabled.vi"("error in (no error)"=w629, "output enabled"=w578, "channel name"="1", "instrument handle"=w630) -> ("error out"=w672:errorcluster, "instrument handle out"=w673:refnum<k15>)  [unwired: 6 in]
        n373 = call <instrlib>:"niDCPower Configure Output Enabled.vi"("error in (no error)"=w618, "output enabled"=w578, "channel name"="0", "instrument handle"=w619) -> ("error out"=w610:errorcluster, "instrument handle out"=w611:refnum<k15>)  [unwired: 6 in]
        n374 = call <instrlib>:"niDCPower Configure Output Enabled.vi"("error in (no error)"=w606, "output enabled"=w578, "channel name"="2", "instrument handle"=w605) -> ("error out"=w601:errorcluster, "instrument handle out"=w600:refnum<k15>)  [unwired: 6 in]
        n375 = call <instrlib>:"niDCPower Measure.vi"("error in (no error)"=w671, "measurement type"=w583, "channel name"="0", "instrument handle"=w670) -> ("measurement"=→"ADC_cur":dbl, "instrument handle out"=w623:refnum<k15>)  [unwired: 5 in, 1 out]
        n376 = call <instrlib>:"niDCPower Measure.vi"("error in (no error)"=w672, "measurement type"=w583, "channel name"="1", "instrument handle"=w673) -> ("measurement"=→"STAB_cur":dbl)  [unwired: 5 in, 2 out]
        n377 = call <instrlib>:"niDCPower Measure.vi"("error in (no error)"=w601, "measurement type"=w583, "channel name"="2", "instrument handle"=w600) -> ("measurement"=→"-15_cur":dbl)  [unwired: 5 in, 2 out]
        n378 = call <instrlib>:"niDCPower Measure.vi"("error in (no error)"=w687, "measurement type"=w583, "channel name"="1", "instrument handle"=w680) -> ("measurement"=→"RD_cur":dbl, "instrument handle out"=w622:refnum<k15>)  [unwired: 5 in, 1 out]
        n379 = call <instrlib>:"niDCPower Measure.vi"("error in (no error)"=w682, "measurement type"=w583, "channel name"="2", "instrument handle"=w681) -> ("measurement"=→"PH_LOW_cur":dbl)  [unwired: 5 in, 2 out]
        n380 = call <instrlib>:"niDCPower Measure.vi"("error in (no error)"=w610, "measurement type"=w583, "channel name"="0", "instrument handle"=w611) -> ("measurement"=→"4V_cur":dbl)  [unwired: 5 in, 2 out]
        n381 = call <instrlib>:"niDCPower Measure.vi"("error in (no error)"=w684, "measurement type"=w583, "channel name"="0", "instrument handle"=w683) -> ("measurement"=→"1V_cur":dbl, "instrument handle out"=w621:refnum<k15>)  [unwired: 5 in, 1 out]
        n382 = call <instrlib>:"niDCPower Measure.vi"("error in (no error)"=w685, "measurement type"=w583, "channel name"="1", "instrument handle"=w686) -> ("measurement"=→"VDD_cur":dbl)  [unwired: 5 in, 2 out]
        n383 = call <instrlib>:"niDCPower Measure.vi"("error in (no error)"=w586, "measurement type"=w583, "channel name"="2", "instrument handle"=w585) -> ("measurement"=→"PS_LOW_cur":dbl)  [unwired: 5 in, 2 out]
      }
    }
    n384 = Wait (ms)(milliseconds to wait=u32 1) -> ()  [unwired: 1 out]
  }
  n385 = while {
    tunnel: w1 -> [w704]
    shift-right: ["文韧 世男!"] -> _
    shift-left: _ -> [w700]
    stop <- w705 stop-if-true
    # "Запрос кадра"
    n386 = local read "Линейки"() -> (w703:bool)
    n387 = local read "Питание"() -> (w702:bool)
    n388 = Greater?(x="文韧 世男!", y=w700) -> (0:w696:bool)
    n389 = Or(x=w696, y="НЕПРЕРЫВНО") -> (x .or. y?=w698:bool)
    n390 = Compound Arithmetic op=AND(w698, w703, w702) -> (w701:bool)
    n391 = case shown="True" w701 {
      tunnel: w704 -> [_ w707]
      frame False {
        n392 = Wait (ms)(milliseconds to wait=u32 1) -> ()  [unwired: 1 out]
      }
      frame True {
        n393 = stacked-sequence {
          seq-local: [_ w719 _ _ _ _] -> [_ _ w789 _ _ _]
          seq-local: [_ _ w799 _ _ _] -> [_ _ _ w831 _ _]
          seq-local: [_ _ _ w830 _ _] -> [_ _ _ _ w835 _]
          tunnel: w707 -> [w709 w720 _ _ _ _]
          frame #0 {
            n394 = xnode "Invoke Method"("FPGA VI Reference In"=w709, "Number of Elements"=u32 0, "Timeout (ms)"=0) -> ("FPGA VI Reference Out"=w714:refnum<k20>, "Elements Remaining"=w713:u32)  [unwired: 1 in, 2 out]
            n395 = local write "БД"(0 ("БД")) -> ()
            n396 = xnode "Invoke Method"("FPGA VI Reference In"=w714, "Number of Elements"=w713, "Timeout (ms)"=0) -> ()  [unwired: 1 in, 4 out]
          }
          frame #1 {
            n397 = for {
              N: "Усреднение" -> [_]
              tunnel: w720 -> [w728]
              shift-right: [w725] -> w717
              shift-left: u64[] array[125550 elements] -> [w726]
              n398 = stacked-sequence {
                seq-local: [_ w733 _ _] -> [_ _ w745 _]
                tunnel: w728 -> [w730 w732 w739 _]
                tunnel: [_ _ w741 _] -> w727
                frame #0 {
                  n399 = xnode "Read/Write Control"("FPGA VI Reference In"=w730, "Кадр в FIFO"=TRUE) -> ()  [unwired: 1 in, 2 out]
                  n400 = Wait (ms)(milliseconds to wait=u32 300) -> ()  [unwired: 1 out]
                }
                frame #1 {
                  n401 = xnode "Invoke Method"("FPGA VI Reference In"=w732, "Number of Elements"=u32 0, "Timeout (ms)"=0) -> ("FPGA VI Reference Out"=w735:refnum<k20>, "Elements Remaining"=w734:u32)  [unwired: 1 in, 2 out]
                  n402 = xnode "Invoke Method"("FPGA VI Reference In"=w735, "Number of Elements"=w734, "Timeout (ms)"=0) -> ("Data"=w733:u8[])  [unwired: 1 in, 3 out]
                }
                frame #2 {
                  # "L"
                  # "H"
                  n403 = Decimate 1D Array(w745) -> (w744:u8[], w743:u8[])
                  n404 = for {
                    N: 125550 -> [_]
                    tunnel: w744 -> [w755]
                    tunnel: w743 -> [w754]
                    tunnel: [w746] -> w741 mode=indexing
                    i -> [w753]
                    n405 = Index Array(array=w754, index=w753) -> (element=w751:u8)
                    n406 = Index Array(array=w755, index=w753) -> (element=w752:u8)
                    n407 = To Unsigned Word Integer(number=w751) -> (unsigned 16bit integer=w747:u16)
                    n408 = To Unsigned Word Integer(number=w752) -> (unsigned 16bit integer=w750:u16)
                    n409 = Multiply(x=w750, y=u16 256) -> (x*y=w748:u16)
                    n410 = Add(x=w748, y=w747) -> (x+y=w746:u16)
                  }
                  n411 = xnode "Read/Write Control"("FPGA VI Reference In"=w739, "Кадр в FIFO"=FALSE) -> ()  [unwired: 1 in, 2 out]
                }
                frame #3 {
                  n412 = Wait (ms)(milliseconds to wait=u32 300) -> ()  [unwired: 1 out]
                }
              }
              n413 = Add(x=w727, y=w726) -> (x+y=w725:u64[])
            }
            n414 = local write "FRAME_OK"(FALSE ("FRAME_OK")) -> ()
            n415 = for {
              tunnel: w717 -> [w724] mode=indexing
              tunnel: "Усреднение" -> [w723]
              tunnel: [w721] -> w719 mode=indexing
              n416 = Divide(x=w724, y=w723) -> (x/y=w722:dbl)
              n417 = To Unsigned Word Integer(number=w722) -> (unsigned 16bit integer=w721:u16)
            }
          }
          frame #2 {
            w763 = 400 ("length")
            w764 = 180 ("length")
            w794 = 5 ("length")
            w793 = 5 ("length")
            n418 = Multiply(x=w764, y=w763) -> (x*y=w767:i32)
            n419 = Multiply(x=w789, y="ISO") -> (x*y=w788:dbl[])
            n420 = To Unsigned Word Integer(number=w788) -> (unsigned 16bit integer=w787:u16[])
            n421 = for {
              N: 270 -> [_]
              tunnel: [w826] -> w758 mode=indexing
              shift-right: [w825] -> _
              shift-left: w787 -> [w829]
              n422 = Delete From Array(array=w829, length=465, index=0) -> (deleted portion=w826:u16[], array with subset deleted=w825:u16[])
            }
            "FRAME" <- w758
            n423 = Array Subset(array=w758, index (row)=55 ("index"), length (row)=w764, index (col)=45 ("index"), length (col)=w763) -> (w761:u16[][])
            n424 = Reshape Array(w761, w767) -> (w760:u16[])
            n425 = for {
              tunnel: w758 -> [w821] mode=indexing
              tunnel: [w820] -> w799 mode=indexing
              n426 = for {
                N: 465 -> [_]
                tunnel: [w824] -> w820 mode=indexing
                tunnel: w821 -> [w823] mode=indexing
                n427 = Bundle(w823, w823, w823, w823) -> (w824:cluster{u16, u16, u16, u16})  [unwired: 1 in]
              }
            }
            "OUT" <- w799
            n428 = for {
              tunnel: w760 -> [w803] mode=indexing
              shift-right: [w801] -> w759
              shift-left: u64 0 -> [w802]
              n429 = Add(x=w803, y=w802) -> (x+y=w801:u64)
            }
            n430 = Divide(x=w759, y=w767) -> (x/y=w757:dbl)
            n431 = Array Subset(array=w758, index (row)=50 ("index"), length (row)=190 ("length"), index (col)=39 ("index"), length (col)=414 ("length")) -> (w771:u16[][])
            n432 = Multiply(x=w793, y=w794) -> (x*y=w778:i32)
            n433 = Array Subset(array=w758, index (row)=5 ("index"), length (row)=w793, index (col)=5 ("index"), length (col)=w794) -> (w796:u16[][])
            n434 = Array Subset(array=w758, index (row)=5 ("index"), length (row)=5 ("length"), index (col)=5 ("index"), length (col)=5 ("length")) -> (w785:u16[][])
            n435 = Reshape Array(w796, w778) -> (w797:u16[])
            n436 = Reshape Array(w785, w778) -> (w781:u16[])
            n437 = Multiply(x=5.0, y=w757) -> (x*y=w768:dbl)
            n438 = for {
              tunnel: w771 -> [w805] mode=indexing
              tunnel: w768 -> [w804]
              n439 = for {
                tunnel: w805 -> [w808] mode=indexing
                tunnel: w804 -> [w806]
                n440 = Greater Or Equal?(x=w808, y=w806) -> (x >= y?=w807:bool)
                n441 = case shown="True" w807 {
                  frame False {
                  }
                  frame True {
                    n442 = local read "БД"() -> (w810:i32)
                    n443 = Increment(x=w810) -> (x+1=→"БД":i32)
                  }
                }
              }
            }
            n444 = for {
              tunnel: w797 -> [w819] mode=indexing
              shift-right: [w817] -> w798
              shift-left: u64 0 -> [w818]
              n445 = Add(x=w819, y=w818) -> (x+y=w817:u64)
            }
            n446 = Divide(x=w798, y=w778) -> (x/y=w770:dbl)
            "Среднее" <- w770
            n447 = for {
              tunnel: w770 -> [w815]
              tunnel: w781 -> [w816] mode=indexing
              shift-right: [w811] -> w786
              shift-left: 0.0 -> [w813]
              n448 = Subtract(x=w816, y=w815) -> (x-y=w814:dbl)
              n449 = Square(x=w814) -> (x^2=w812:dbl)
              n450 = Add(x=w812, y=w813) -> (x+y=w811:dbl)
            }
            n451 = Divide(x=w786, y=w778) -> (x/y=w777:dbl)
            n452 = Square Root(x=w777) -> (sqrt(x)=→"СКО":dbl)
          }
          frame #3 {
            w832 = T5 6 items=["Grayscale (U8)", "Grayscale (I16)", "Grayscale (SGL)", "Complex (CSG)", "RGB (U32)", "HSL (U32)", "RGB (U64)"] ("Image Type")
            n453 = call "IMAQ Create"("Image Name"="FPZC", "Image Type"=w832) -> ("New Image"=w834:T1)  [unwired: 3 in, 1 out]
            n454 = call "IMAQ ArrayToColorImage"("Image"=w834, "Image Pixels (U64)"=w831) -> ("Image Out"=w830:T1)  [unwired: 3 in, 1 out]
            "Image" <- w830
          }
          frame #4 {
            n455 = case shown="True" "Запись Кадра" {
              tunnel: w835 -> [_ w840]
              frame False {
              }
              frame True {
                w845 = i16 0 ("precision (6)")
                w839 = "_"
                n456 = local read "Между кадрами, мс"() -> (w857:u8)
                n457 = local read "Номер образца"() -> (w851:string)
                n458 = Concatenate Strings("Образец_" ("string"), w851) -> (w846:string)
                n459 = Get Date/Time In Seconds() -> (seconds since 1Jan1904=w854:timestamp)
                n460 = Build Path(base path="Frames", name or relative path=w846) -> (appended path=w850:path)
                n461 = Number To Fractional String(number=w857, width (-)=w845, precision (6)=w845) -> (F-format string=w858:string)  [unwired: 1 in]
                n462 = Format Date/Time String(time format string (%c)="%H.%M.%S", seconds (now)=w854) -> (date/time string=w856:string)  [unwired: 1 in]
                n463 = call <vilib>:"Check if File or Folder Exists.vi"("path"=w850) -> ("file or folder exists?"=w849:bool, "dup path"=w848:path)  [unwired: 8 in, 1 out]
                n464 = case shown="False" w849 {
                  tunnel: w848 -> [w861 w862]
                  tunnel: [w860 w862] -> w855
                  frame False {
                    n465 = Create Folder(path (use dialog)=w861) -> (created path=w860:path)  [unwired: 2 in, 2 out]
                  }
                  frame True {
                  }
                }
                n466 = Concatenate Strings(w856, w839, "Тн=" ("string"), w858, "мс_" ("string"), "ПРИМЕЧАНИЕ", w839, "Какая фотка?", ".tiff" ("element")) -> (w852:string)
                n467 = Build Path(base path=w855, name or relative path=w852) -> (appended path=w853:path)
                n468 = call-poly "IMAQ Write File 2"("File Path"=w853, "Image"=w840) -> ()  [unwired: 8 in, 2 out]
              }
            }
          }
          frame #5 {
            "FRAME_OK" <- TRUE
          }
        }
      }
    }
    n469 = local read "Стоп"() -> (w705:bool)
  }
  n470 = while {
    tunnel: w1 -> [w869]
    shift-right: ["Прошить АЦП"] -> _
    shift-left: FALSE -> [w868]
    stop <- w870 stop-if-true
    n471 = Greater?(x="Прошить АЦП", y=w868) -> (0:w866:bool)
    n472 = local read "Питание"() -> (w864:bool)
    n473 = And(x=w864, y=w866) -> (x .and. y?=w865:bool)
    n474 = case shown="True" w865 {
      tunnel: w869 -> [_ w872]
      frame False {
        n475 = Wait (ms)(milliseconds to wait=u32 1) -> ()  [unwired: 1 out]
      }
      frame True {
        n476 = stacked-sequence {
          tunnel: w872 -> [w898 w938 w952 w981 w1025 w1035 w1060 w1093 _]
          frame #0 {
            w894 = TRUE ("element")
            w895 = FALSE
            # "8"
            # "0"
            # "Configuration"
            n477 = xnode "Read/Write Control"("FPGA VI Reference In"=w898, "Enum"=T6."Configuration") -> ("FPGA VI Reference Out"=w885:refnum<k20>)  [unwired: 1 in, 1 out]
            n478 = xnode "Read/Write Control"("FPGA VI Reference In"=w875, "Read(T)/Write(F)"=TRUE) -> ("FPGA VI Reference Out"=w881:refnum<k20>, "error out"=w880:errorcluster)  [unwired: 1 in]
            n479 = case shown="\"3CH\", Default" "3CH/1CH" {
              tunnel: [TRUE FALSE] -> w893
              frame "3CH", Default {
              }
              frame "1CH" {
              }
            }
            n480 = case shown="\"4V\"" "2/4 V" {
              tunnel: [FALSE TRUE] -> w891
              frame "2V", Default {
              }
              frame "4V" {
              }
            }
            n481 = xnode "Read/Write Control"("FPGA VI Reference In"=w885, "Read(T)/Write(F)"=FALSE) -> ("FPGA VI Reference Out"=w883:refnum<k20>)  [unwired: 1 in, 1 out]
            n482 = flat-sequence {
              tunnel: w881 -> [w910]
              tunnel: w880 -> [w909]
              tunnel: [w908] -> w879
              tunnel: [w907] -> w878
              frame #0 {
                n483 = xnode "Read/Write Control"("FPGA VI Reference In"=w910, "error in"=w909, "Конфигурация"=TRUE) -> ("FPGA VI Reference Out"=w908:refnum<k20>, "error out"=w907:errorcluster)
                n484 = Wait (ms)(milliseconds to wait=u32 10) -> ()  [unwired: 1 out]
              }
            }
            n485 = Build Array(w895, w895, w895, w894, w894, w893, w894, w891, FALSE) -> (w896:bool[])
            n486 = Reverse 1D Array(array=w896) -> (reversed array=w888:bool[])
            n487 = xnode "Read/Write Control"("FPGA VI Reference In"=w883, "Write Data"=w888) -> ("FPGA VI Reference Out"=w887:refnum<k20>)  [unwired: 1 in, 1 out]
            n488 = flat-sequence {
              tunnel: w879 -> [w904]
              tunnel: w878 -> [w903]
              tunnel: [w901] -> w877
              tunnel: [w900] -> w876
              frame #0 {
                n489 = xnode "Read/Write Control"("FPGA VI Reference In"=w904, "error in"=w903, "Конфигурация"=FALSE) -> ("FPGA VI Reference Out"=w901:refnum<k20>, "error out"=w900:errorcluster)
                n490 = Wait (ms)(milliseconds to wait=u32 10) -> ()  [unwired: 1 out]
              }
            }
            n491 = flat-sequence {
              tunnel: w887 -> [w918]
              tunnel: [w916] -> w886
              frame #0 {
                n492 = xnode "Read/Write Control"("FPGA VI Reference In"=w918, "Конфигурация"=TRUE) -> ("FPGA VI Reference Out"=w916:refnum<k20>)  [unwired: 1 in, 1 out]
                n493 = Wait (ms)(milliseconds to wait=u32 10) -> ()  [unwired: 1 out]
              }
            }
            n494 = local write "АЦП прошит!"(FALSE ("АЦП прошит!")) -> ()
            n495 = xnode "Read/Write Control"("FPGA VI Reference In"=w877, "error in"=w876) -> ("READ"=→"Configuration":bool[])  [unwired: 2 out]
            n496 = flat-sequence {
              tunnel: w886 -> [w914]
              tunnel: [w912] -> w875
              frame #0 {
                n497 = xnode "Read/Write Control"("FPGA VI Reference In"=w914, "Конфигурация"=FALSE) -> ("FPGA VI Reference Out"=w912:refnum<k20>)  [unwired: 1 in, 1 out]
                n498 = Wait (ms)(milliseconds to wait=u32 10) -> ()  [unwired: 1 out]
              }
            }
          }
          frame #1 {
            # "GREEN_OFFSET"
            n499 = case shown="\"-\", Default" "+/- OUT1" {
              tunnel: [TRUE FALSE] -> w925
              frame "-", Default {
              }
              frame "+" {
              }
            }
            n500 = Quotient & Remainder(x="Смещение, до 300_OUT1", y=1.171875) -> (floor(x/y)=w930:dbl)  [unwired: 1 out]
            n501 = xnode "Read/Write Control"("FPGA VI Reference In"=w938, "Enum"=T6."GREEN OFF" ("OFFSET")) -> ("FPGA VI Reference Out"=w937:refnum<k20>, "error out"=w936:errorcluster)  [unwired: 1 in]
            n502 = Subtract(x=w930, y=1.0) -> (x-y=w927:dbl)
            n503 = To Unsigned Byte Integer(number=w927) -> (unsigned 8bit integer=w926:u8)
            n504 = xnode "Read/Write Control"("FPGA VI Reference In"=w937, "error in"=w936, "Read(T)/Write(F)"=FALSE) -> ("FPGA VI Reference Out"=w935:refnum<k20>)  [unwired: 1 out]
            n505 = Number To Boolean Array(number=w926) -> (Boolean array=w924:bool[])
            n506 = Reverse 1D Array(array=w924) -> (reversed array=w923:bool[])
            n507 = Build Array (concatenate)(w925, w923) -> (w928:bool[])
            n508 = xnode "Read/Write Control"("FPGA VI Reference In"=w935, "Write Data"=w928) -> ("FPGA VI Reference Out"=w940:refnum<k20>)  [unwired: 1 in, 1 out]
            n509 = flat-sequence {
              tunnel: w940 -> [w951]
              tunnel: [w949] -> w939
              frame #0 {
                n510 = xnode "Read/Write Control"("FPGA VI Reference In"=w951, "Конфигурация"=TRUE) -> ("FPGA VI Reference Out"=w949:refnum<k20>)  [unwired: 1 in, 1 out]
                n511 = Wait (ms)(milliseconds to wait=u32 10) -> ()  [unwired: 1 out]
              }
            }
            n512 = flat-sequence {
              tunnel: w939 -> [w947]
              tunnel: [w945] -> _
              frame #0 {
                n513 = xnode "Read/Write Control"("FPGA VI Reference In"=w947, "Конфигурация"=FALSE) -> ("FPGA VI Reference Out"=w945:refnum<k20>)  [unwired: 1 in, 1 out]
                n514 = Wait (ms)(milliseconds to wait=u32 10) -> ()  [unwired: 1 out]
              }
            }
          }
          frame #2 {
            # "RED_OFFSET"
            n515 = case shown="\"-\", Default" "+/- OUT4" {
              tunnel: [TRUE FALSE] -> w968
              frame "-", Default {
              }
              frame "+" {
              }
            }
            n516 = Quotient & Remainder(x="Смещение, до 300_OUT4", y=1.171875) -> (floor(x/y)=w963:dbl)  [unwired: 1 out]
            n517 = xnode "Read/Write Control"("FPGA VI Reference In"=w952, "Enum"=T6."RED OFF" ("OFFSET")) -> ("FPGA VI Reference Out"=w959:refnum<k20>, "error out"=w960:errorcluster)  [unwired: 1 in]
            n518 = Subtract(x=w963, y=1.0) -> (x-y=w966:dbl)
            n519 = To Unsigned Byte Integer(number=w966) -> (unsigned 8bit integer=w967:u8)
            n520 = xnode "Read/Write Control"("FPGA VI Reference In"=w959, "error in"=w960, "Read(T)/Write(F)"=FALSE) -> ("FPGA VI Reference Out"=w961:refnum<k20>)  [unwired: 1 out]
            n521 = Number To Boolean Array(number=w967) -> (Boolean array=w969:bool[])
            n522 = Reverse 1D Array(array=w969) -> (reversed array=w970:bool[])
            n523 = Build Array (concatenate)(w968, w970) -> (w965:bool[])
            n524 = xnode "Read/Write Control"("FPGA VI Reference In"=w961, "Write Data"=w965) -> ("FPGA VI Reference Out"=w957:refnum<k20>)  [unwired: 1 in, 1 out]
            n525 = flat-sequence {
              tunnel: w957 -> [w980]
              tunnel: [w978] -> w958
              frame #0 {
                n526 = xnode "Read/Write Control"("FPGA VI Reference In"=w980, "Конфигурация"=TRUE) -> ("FPGA VI Reference Out"=w978:refnum<k20>)  [unwired: 1 in, 1 out]
                n527 = Wait (ms)(milliseconds to wait=u32 10) -> ()  [unwired: 1 out]
              }
            }
            n528 = flat-sequence {
              tunnel: w958 -> [w976]
              tunnel: [w974] -> _
              frame #0 {
                n529 = xnode "Read/Write Control"("FPGA VI Reference In"=w976, "Конфигурация"=FALSE) -> ("FPGA VI Reference Out"=w974:refnum<k20>)  [unwired: 1 in, 1 out]
                n530 = Wait (ms)(milliseconds to wait=u32 10) -> ()  [unwired: 1 out]
              }
            }
          }
          frame #3 {
            # "BLUE_OFFSET"
            n531 = case shown="\"-\", Default" "+/- OUT2" {
              tunnel: [TRUE FALSE] -> w997
              frame "-", Default {
              }
              frame "+" {
              }
            }
            n532 = Quotient & Remainder(x="Смещение, до 300_OUT2", y=1.171875) -> (floor(x/y)=w992:dbl)  [unwired: 1 out]
            n533 = xnode "Read/Write Control"("FPGA VI Reference In"=w981, "Enum"=T6."BLUE OFF" ("OFFSET")) -> ("FPGA VI Reference Out"=w988:refnum<k20>, "error out"=w989:errorcluster)  [unwired: 1 in]
            n534 = Subtract(x=w992, y=1.0) -> (x-y=w995:dbl)
            n535 = To Unsigned Byte Integer(number=w995) -> (unsigned 8bit integer=w996:u8)
            n536 = xnode "Read/Write Control"("FPGA VI Reference In"=w988, "error in"=w989, "Read(T)/Write(F)"=FALSE) -> ("FPGA VI Reference Out"=w990:refnum<k20>)  [unwired: 1 out]
            n537 = Number To Boolean Array(number=w996) -> (Boolean array=w998:bool[])
            n538 = Reverse 1D Array(array=w998) -> (reversed array=w999:bool[])
            n539 = Build Array (concatenate)(w997, w999) -> (w994:bool[])
            n540 = xnode "Read/Write Control"("FPGA VI Reference In"=w990, "Write Data"=w994) -> ("FPGA VI Reference Out"=w986:refnum<k20>)  [unwired: 1 in, 1 out]
            n541 = flat-sequence {
              tunnel: w986 -> [w1009]
              tunnel: [w1007] -> w987
              frame #0 {
                n542 = xnode "Read/Write Control"("FPGA VI Reference In"=w1009, "Конфигурация"=TRUE) -> ("FPGA VI Reference Out"=w1007:refnum<k20>)  [unwired: 1 in, 1 out]
                n543 = Wait (ms)(milliseconds to wait=u32 10) -> ()  [unwired: 1 out]
              }
            }
            n544 = flat-sequence {
              tunnel: w987 -> [w1005]
              tunnel: [w1003] -> _
              frame #0 {
                n545 = xnode "Read/Write Control"("FPGA VI Reference In"=w1005, "Конфигурация"=FALSE) -> ("FPGA VI Reference Out"=w1003:refnum<k20>)  [unwired: 1 in, 1 out]
                n546 = Wait (ms)(milliseconds to wait=u32 10) -> ()  [unwired: 1 out]
              }
            }
          }
          frame #4 {
            w1020 = FALSE
            # "GREEN PGA"
            n547 = Decrement(x="Усиление (до 6)_OUT1") -> (x-1=w1012:u8)
            n548 = Multiply(x=w1012, y=378) -> (x*y=w1014:i32)
            n549 = Multiply(x="Усиление (до 6)_OUT1", y=5) -> (x*y=w1017:i32)
            n550 = xnode "Read/Write Control"("FPGA VI Reference In"=w1025, "Enum"=T6."GREEN PGA" ("PGA")) -> ("FPGA VI Reference Out"=w1023:refnum<k20>)  [unwired: 1 in, 1 out]
            n551 = Divide(x=w1014, y=w1017) -> (x/y=w1018:dbl)
            n552 = Number To Boolean Array(number=w1018) -> (Boolean array=w1011:bool[])
            n553 = xnode "Read/Write Control"("FPGA VI Reference In"=w1023, "Read(T)/Write(F)"=FALSE) -> ("FPGA VI Reference Out"=w1022:refnum<k20>)  [unwired: 1 in, 1 out]
            n554 = Build Array (concatenate)(w1020, w1020, w1020, w1011) -> (w1019:bool[])
            n555 = xnode "Read/Write Control"("FPGA VI Reference In"=w1022, "Write Data"=w1019) -> ("FPGA VI Reference Out"=w1024:refnum<k20>)  [unwired: 1 in, 1 out]
            n556 = flat-sequence {
              tunnel: [w1033] -> w1026
              tunnel: w1024 -> [w1032]
              frame #0 {
                n557 = xnode "Read/Write Control"("FPGA VI Reference In"=w1032, "Конфигурация"=TRUE) -> ("FPGA VI Reference Out"=w1033:refnum<k20>)  [unwired: 1 in, 1 out]
                n558 = Wait (ms)(milliseconds to wait=u32 10) -> ()  [unwired: 1 out]
              }
            }
            n559 = flat-sequence {
              tunnel: w1026 -> [w1030]
              tunnel: [w1028] -> _
              frame #0 {
                n560 = xnode "Read/Write Control"("FPGA VI Reference In"=w1030, "Конфигурация"=FALSE) -> ("FPGA VI Reference Out"=w1028:refnum<k20>)  [unwired: 1 in, 1 out]
                n561 = Wait (ms)(milliseconds to wait=u32 10) -> ()  [unwired: 1 out]
              }
            }
          }
          frame #5 {
            w1038 = FALSE
            # "BLUE PGA"
            n562 = Decrement(x="Усиление (до 6)_OUT2") -> (x-1=w1042:u8)
            n563 = Multiply(x=w1042, y=378) -> (x*y=w1043:i32)
            n564 = Multiply(x="Усиление (до 6)_OUT2", y=5) -> (x*y=w1045:i32)
            n565 = xnode "Read/Write Control"("FPGA VI Reference In"=w1035, "Enum"=T6."BLUE PGA" ("PGA")) -> ("FPGA VI Reference Out"=w1049:refnum<k20>)  [unwired: 1 in, 1 out]
            n566 = Divide(x=w1043, y=w1045) -> (x/y=w1046:dbl)
            n567 = Number To Boolean Array(number=w1046) -> (Boolean array=w1041:bool[])
            n568 = xnode "Read/Write Control"("FPGA VI Reference In"=w1049, "Read(T)/Write(F)"=FALSE) -> ("FPGA VI Reference Out"=w1048:refnum<k20>)  [unwired: 1 in, 1 out]
            n569 = Build Array (concatenate)(w1038, w1038, w1038, w1041) -> (w1047:bool[])
            n570 = xnode "Read/Write Control"("FPGA VI Reference In"=w1048, "Write Data"=w1047) -> ("FPGA VI Reference Out"=w1050:refnum<k20>)  [unwired: 1 in, 1 out]
            n571 = flat-sequence {
              tunnel: [w1058] -> w1051
              tunnel: w1050 -> [w1057]
              frame #0 {
                n572 = xnode "Read/Write Control"("FPGA VI Reference In"=w1057, "Конфигурация"=TRUE) -> ("FPGA VI Reference Out"=w1058:refnum<k20>)  [unwired: 1 in, 1 out]
                n573 = Wait (ms)(milliseconds to wait=u32 10) -> ()  [unwired: 1 out]
              }
            }
            n574 = flat-sequence {
              tunnel: w1051 -> [w1055]
              tunnel: [w1053] -> _
              frame #0 {
                n575 = xnode "Read/Write Control"("FPGA VI Reference In"=w1055, "Конфигурация"=FALSE) -> ("FPGA VI Reference Out"=w1053:refnum<k20>)  [unwired: 1 in, 1 out]
                n576 = Wait (ms)(milliseconds to wait=u32 10) -> ()  [unwired: 1 out]
              }
            }
          }
          frame #6 {
            w1071 = FALSE
            # "RED PGA"
            n577 = Decrement(x="Усиление (до 6)_OUT4") -> (x-1=w1063:u8)
            n578 = Multiply(x=w1063, y=378) -> (x*y=w1065:i32)
            n579 = Multiply(x="Усиление (до 6)_OUT4", y=5) -> (x*y=w1068:i32)
            n580 = xnode "Read/Write Control"("FPGA VI Reference In"=w1060, "Enum"=T6."RED PGA" ("PGA")) -> ("FPGA VI Reference Out"=w1074:refnum<k20>)  [unwired: 1 in, 1 out]
            n581 = Divide(x=w1065, y=w1068) -> (x/y=w1069:dbl)
            n582 = Number To Boolean Array(number=w1069) -> (Boolean array=w1062:bool[])
            n583 = xnode "Read/Write Control"("FPGA VI Reference In"=w1074, "Read(T)/Write(F)"=FALSE) -> ("FPGA VI Reference Out"=w1073:refnum<k20>)  [unwired: 1 in, 1 out]
            n584 = Build Array (concatenate)(w1071, w1071, w1071, w1062) -> (w1070:bool[])
            n585 = xnode "Read/Write Control"("FPGA VI Reference In"=w1073, "Write Data"=w1070) -> ("FPGA VI Reference Out"=w1075:refnum<k20>)  [unwired: 1 in, 1 out]
            n586 = flat-sequence {
              tunnel: [w1083] -> w1076
              tunnel: w1075 -> [w1082]
              frame #0 {
                n587 = xnode "Read/Write Control"("FPGA VI Reference In"=w1082, "Конфигурация"=TRUE) -> ("FPGA VI Reference Out"=w1083:refnum<k20>)  [unwired: 1 in, 1 out]
                n588 = Wait (ms)(milliseconds to wait=u32 10) -> ()  [unwired: 1 out]
              }
            }
            n589 = flat-sequence {
              tunnel: w1076 -> [w1080]
              tunnel: [w1078] -> _
              frame #0 {
                n590 = xnode "Read/Write Control"("FPGA VI Reference In"=w1080, "Конфигурация"=FALSE) -> ("FPGA VI Reference Out"=w1078:refnum<k20>)  [unwired: 1 in, 1 out]
                n591 = Wait (ms)(milliseconds to wait=u32 10) -> ()  [unwired: 1 out]
              }
            }
          }
          frame #7 {
            # "MUX"
            n592 = xnode "Read/Write Control"("FPGA VI Reference In"=w1093, "Enum"=T6."MUX") -> ("FPGA VI Reference Out"=w1087:refnum<k20>)  [unwired: 1 in, 1 out]
            n593 = case shown="\"OUT1\", Default" "Какой канал?" {
              tunnel: [bool[] [FALSE, TRUE, FALSE, TRUE, FALSE, FALSE, FALSE, FALSE, FALSE] ("MUX_register") bool[] [FALSE, TRUE, FALSE, FALSE, TRUE, FALSE, FALSE, FALSE, FALSE] ("MUX_register") bool[] [FALSE, TRUE, TRUE, FALSE, FALSE, FALSE, FALSE, FALSE, FALSE] ("MUX_register")] -> w1085
              frame "OUT1", Default {
              }
              frame "OUT2" {
              }
              frame "OUT4" {
              }
            }
            n594 = xnode "Read/Write Control"("FPGA VI Reference In"=w1087, "Read(T)/Write(F)"=FALSE) -> ("FPGA VI Reference Out"=w1089:refnum<k20>)  [unwired: 1 in, 1 out]
            n595 = xnode "Read/Write Control"("FPGA VI Reference In"=w1089, "Write Data"=w1085) -> ("FPGA VI Reference Out"=w1090:refnum<k20>)  [unwired: 1 in, 1 out]
            n596 = flat-sequence {
              tunnel: [w1103] -> w1091
              tunnel: w1090 -> [w1102]
              frame #0 {
                n597 = xnode "Read/Write Control"("FPGA VI Reference In"=w1102, "Конфигурация"=TRUE) -> ("FPGA VI Reference Out"=w1103:refnum<k20>)  [unwired: 1 in, 1 out]
                n598 = Wait (ms)(milliseconds to wait=u32 10) -> ()  [unwired: 1 out]
              }
            }
            n599 = flat-sequence {
              tunnel: w1091 -> [w1100]
              tunnel: [w1098] -> _
              frame #0 {
                n600 = xnode "Read/Write Control"("FPGA VI Reference In"=w1100, "Конфигурация"=FALSE) -> ("FPGA VI Reference Out"=w1098:refnum<k20>)  [unwired: 1 in, 1 out]
                n601 = Wait (ms)(milliseconds to wait=u32 10) -> ()  [unwired: 1 out]
              }
            }
          }
          frame #8 {
            "АЦП прошит!" <- TRUE ("АЦП прошит!")
          }
        }
      }
    }
    n602 = local read "Стоп"() -> (w870:bool)
  }
  n603 = while {
    tunnel: w1 -> [w1141]
    tunnel: [w1140] -> w4
    stop <- w1139 stop-if-true
    # "Общие настройки"
    n604 = local read "Питание"() -> (w1143:bool)
    n605 = case shown="\"MAX\"" "Частота?" {
      tunnel: ["CDS1_2" u8 6 ("CDS1_2")] -> w1125
      tunnel: ["CDS1_1" u8 2 ("CDS1_1")] -> w1124
      tunnel: ["CDS2_2" u8 6 ("CDS2_2")] -> w1123
      tunnel: ["CDS2_1" u8 0 ("CDS2_1")] -> w1122
      tunnel: ["ADC_2" u8 7 ("ADC_2")] -> w1121
      tunnel: ["ADC_1" u8 2 ("ADC_1")] -> w1120
      tunnel: ["RG_2" u8 2 ("RG_2")] -> w1119
      tunnel: ["RG1" u8 1 ("RG1")] -> w1118
      tunnel: ["PH2_2" u8 5 ("PH2_2")] -> w1117
      tunnel: ["PH2_1" u8 1 ("PH2_1")] -> w1116
      tunnel: ["PH1_2" u8 5 ("PH1_2")] -> w1115
      tunnel: ["PH1_1" u8 1 ("PH1_1")] -> w1114
      tunnel: ["HOR" u16 465 ("HOR")] -> w1113
      tunnel: ["8" u8 8 ("8")] -> w1112
      tunnel: ["LOW" u8 2 ("LOW")] -> w1111
      tunnel: ["HIGH" u8 7 ("HIGH")] -> w1110
      frame "MIN", Default {
      }
      frame "MAX" {
      }
    }
    n606 = And(x="Линейки", y=w1143) -> (x .and. y?=w1137:bool)
    n607 = local read "Стоп"() -> (w1138:bool)
    n608 = xnode "Read/Write Control"("FPGA VI Reference In"=w1141, "Остановка основного цикла"=w1138, "Линейки"=w1137, "Сколько строк?"="Сколько строк?", "Строка триггер"="Строка триггер", "1163"="1163", "PS1_2"="PS1_2", "PS1_1"="PS1_1", "PS21_1"="PS21_1", "PS21_2"="PS21_2", "PS3_1"="PS3_1", "PS3_2"="PS3_2", "PS41_1"="PS41_1", "PS41_2"="PS41_2", "CDS1_2"=w1125, "CDS1_1"=w1124, "CDS2_2"=w1123, "CDS2_1"=w1122, "ADC_2"=w1121, "ADC_1"=w1120, "RG_2"=w1119, "RG1"=w1118, "PH2_2"=w1117, "PH2_1"=w1116, "PH1_2"=w1115, "PH1_1"=w1114, "HOR"=w1113, "8"=w1112, "LOW"=w1111, "HIGH"=w1110, "Направление бит"=FALSE, "Между кадрами"="Между кадрами, мс") -> ("FPGA VI Reference Out"=w1140:refnum<k20>)  [unwired: 1 in, 1 out]
    n609 = Wait (ms)(milliseconds to wait=u32 1) -> ()  [unwired: 1 out]
    n610 = local read "Стоп"() -> (w1139:bool)
  }
  n611 = call <instrlib>:"niDCPower Close.vi"("instrument handle"=w7) -> ()  [unwired: 10 in, 1 out]
  n612 = xnode "Close FPGA VI Reference"("FPGA VI Reference In"=w4) -> ()  [unwired: 1 in, 1 out]
  n613 = call <instrlib>:"niDCPower Close.vi"("instrument handle"=w8) -> ()  [unwired: 10 in, 1 out]
  n614 = call <instrlib>:"niDCPower Close.vi"("instrument handle"=w9) -> ()  [unwired: 10 in, 1 out]
